vi "Tracker_171213.vi"() -> ()   [LabVIEW 2016]
uses:
  Globaltracker.vi
panel:
  in  "EXPORT 2":enum16{"RAW", "TXT", "CSV"}(ring)
  out "TotalDistanceTraveled":dbl
  out "SegmentsRecalculation":bool[](array[boolean])
  out "ForAnalysisLastRecordingPath":path
  in  "i":i32
  out "NotificationCount":i32=3
  out "Alarm":dbl caption="minutes" format="%#g"
  out "Loadedregions":picture
  out "Mousebackground":picture
  out "OutsideaSegment":dbl[](array[slide]) scale=-1.0..83.73750000001033
  out "InsideaSegment":dbl[](array[slide]) scale=-1.0..83.73750000001033
  out "TtlArray":T1(array[cluster])
  in  "Main TabControl":enum32{"Settings", "Recording", "Analysis"}(tab)
  in  "CageSegmentation":enum32{"Page 1", "Page 2"}(tab)
  out "CageSegmentation":string
  out "AssignedSegments":string
  in  "ListboxOfSegments":i32(listbox)
  in  "Border":enum32{"Page 1", "Page 2"}(tab)
  out "Border":string
  in  "Border":enum16{"8", "6", "5", "4", "3", "2", "1", "0"}(ring) caption="Number of\n segments"
  in  "StartingAngleBorder":u16=40 caption="Starting\n angle" max=360 step=1
  in  "Center":enum32{"Page 1", "Page 2"}(tab)
  in  "Center":enum16{"1", "0"}(ring) caption="Number of\n segments"
  in  "RadiusCenter":u16=40 caption="Radius \n (mm)" max=90
  out "Center":string
  in  "Midfield":enum32{"Page 1", "Page 2"}(tab)
  in  "StartingAngleMidfield":u32=40 caption="Starting\n angle" max=360 step=1
  in  "RadiusMidfield":u16=40 caption="Radius\n (mm)" max=90 step=1
  in  "Midfield":enum16{"4", "3", "2", "1", "0"}(ring) caption="Number of\n segments"
  out "Midfiled":string
  out "SettingsDisplay":picture
  out "?":picture
  in  "KeyboardShortcuts":enum32{"Page 1", "Page 2"}(tab)
  out "KeyboardShortcuts":string
  out "_Assigning Buttons_":bool
  in  "KeyBoardShortCuts":bool
  in  "Notifications":enum32{"Page 1", "Page 2"}(tab)
  out "Notifications":string
  out "Notification":bool
  in  "NotificationsON":bool
  in  "FilterType":enum32{"Page 1", "Page 2"}(tab)
  out "FIlterType":string
  in  "FilterType":enum16{"No filter", "Kalman filter"}(ring)
  in  "PortSelection":enum32{"Page 1", "Page 2"}(tab)
  out "PortSelection":string
  in  "Data Port Selection":refnum<visa-resource-name>="ASRL3::INSTR"
  in  "SAVE":bool
  out "?":picture
  in  "KeyboardShortcuts":enum32{"Page 1", "Page 2"}(tab)
  in  "SegmentsMulticolumnListbox":i32(listbox)
  out "KeyboardShortcuts":string
  out "Notification":bool
  out "RecordingDisplay":picture
  in  "Cage Segments":enum32{"Page 1", "Page 2"}(tab)
  out "Segments(s)":dbl[](array[slide]) scale=-1.0..4.437500000000029
  out "Segments":bool[](array[boolean])
  out "1":string
  out "2":string
  out "3":string
  out "4":string
  out "5":string
  out "6":string
  out "7":string
  out "8":string
  out "9":string
  out "10\n10":string
  out "11":string
  out "12":string
  out "13":string
  out "CageSegments":string
  in  "Cage orientation swap":bool caption="Swap coords"
  in  "RecordingTab":enum32{"Page 1", "Page 2"}(tab)
  in  "Stop Button":bool
  in  "Start":bool
  in  "Trace length (s)":dbl(slide) scale=0.0..10.0
  in  "DisplaySegments":enum32{"Page 1", "Page 2"}(tab)
  in  "DisplaySegments":bool caption="Display Segments"
  out "DisplaySegments":string
  in  "CurrentDistanceTraveled":enum32{"Page 1", "Page 2"}(tab)
  out "Current distance\n traveled (m)":dbl(slide) scale=0.0..8.0
  out "CurrentDistanceTraveled":string
  in  "ElapsedTimeRecording":enum32{"Page 1", "Page 2"}(tab)
  out "Time1":string
  out "Time elapsed":string
  out "ElapsedTimeRecording":string
  out "Mouse speed (cm/s)":dbl(knob) scale=0.0..100.0 scale format="%#_6f"
  out "Mouse speed (cm/s)  2":dbl(graph) caption="Mouse speed plotted vs time"
  in  "LoadRecording":enum32{"Page 1", "Page 2"}(tab)
  out "FileName":string
  out "ProgressBar":u16(slide) scale=0.0..100.0
  in  "LOAD RECORDING":bool
  in  "ElapsedTimePlayback":enum32{"Page 1", "Page 2"}(tab)
  out "Time2":string
  out "ElapsedTimePlayback":string
  out "date/time":string
  in  "PlaybackControl":enum32{"Page 1", "Page 2"}(tab)
  in  "Stop Button":bool
  in  "Start/play":bool
  in  "Skip Back Button":bool
  in  "Seek Back Button":bool
  in  "Seek Forward Button":bool
  in  "Skip Forward Button":bool
  in  "Playback progress (min)":dbl(slide) min=0.0 max=24.0 scale=0.0..1.0
  out "Display Speed":dbl
  out "Playback Speed":string
  in  "RemoveButton":bool
  in  "AddButton":bool
  out "AnalysisDisplay":picture
  out "Mouse Speed plotted vs time":dbl(graph) caption="Mouse Speed Plotted vs Time"
  out "Mouse speed (cm/s)":dbl(knob) scale=0.0..100.0
  in  "DisplayOptions":enum32{"Page 1", "Page 2"}(tab)
  in  "Heat Map":bool
  in  "Trace_length (s)":dbl(slide) scale=0.0..10.0
  in  "FullTrack":bool caption="Full Track"
  in  "SegmentsOn":bool caption="Segments"
  out "DisplayOptions":string
  in  "Statistics":enum32{"Page 1", "Page 2"}(tab)
  out "Current Distance\n Traveled (m)":dbl(slide) scale=0.0..1.0 scale format="%#_6f"
  out "Total Distance Traveled (m)":dbl
  out "Average Speed (cm/s)":dbl
  out "TTL":bool
  out "Statitics":string
  in  "EXIT":bool
  out "index":i32
  out "?":picture
  in  "TimeSpentinEachSegment":enum32{"Page 1", "Page 2"}(tab)
  out "TimeSpentinEachSegment":string
  in  "TimeSpentinEachSegmentMultiListBox":i32(listbox)
  out "Heat-Map":dbl[][](graph)
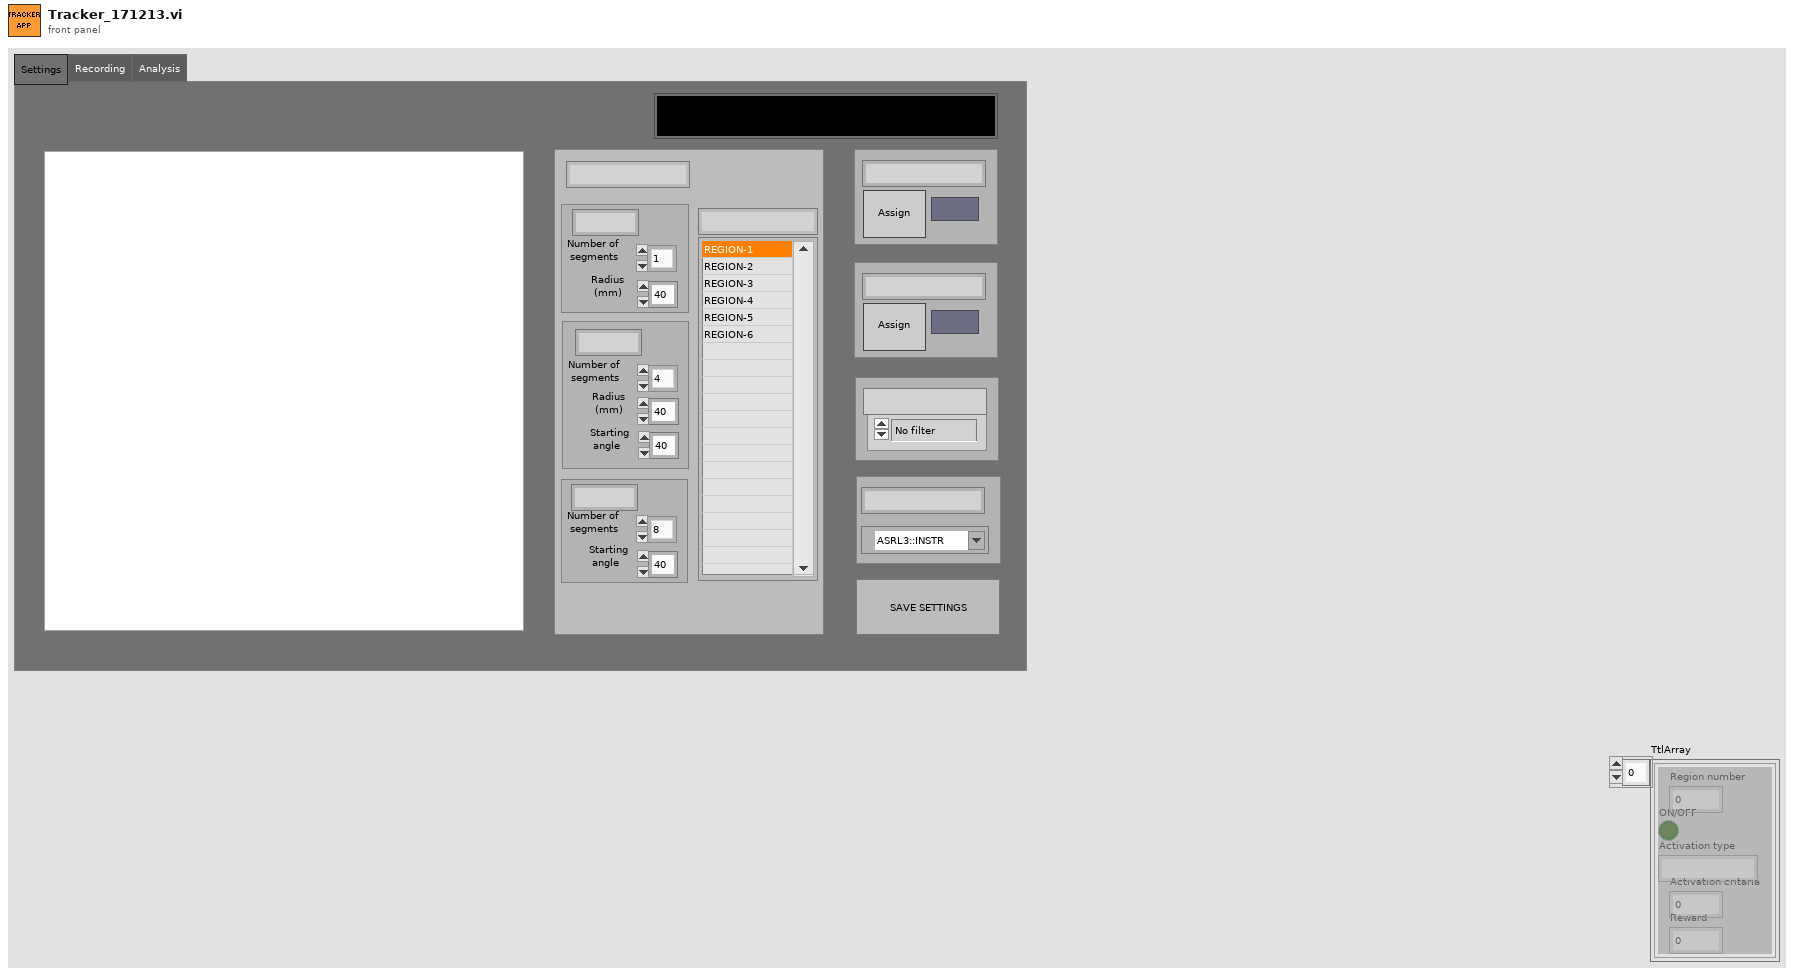
[diagram p1: front panel]
types:
  T1 = cluster{"Region number":i32, "ON/OFF":bool, "Activation type":string, "Activation critaria":i32, "Reward":i32}[]
  T2 = enum16{"No filter", "Kalman filter", "Thresholding"}
  T3 = enum8{"Enabled", "Disabled", "Disabled and Grayed Out"}
  T4 = cluster{"Starting degree of walll":u16, "RewardSystem-ON/OFF":bool, "Image Name":string, "Starting degree of walll":u16, "Starting degree of walll":u16}
  T5 = cluster{"Starting degree of walll":u16, "RewardSystem-ON/OFF":bool, "Image Name":string, "Starting degree of walll":u16, "Starting degree of walll":u16}[]
  T6 = cluster{i32, "ON-OFF":bool, "Activation":string, "ActivationCritaria":i32, "TTLActivation":i32}
  T7 = typedef "imagedata.ctl" = cluster{"image type":i32, "image depth":i32, "image":u8[], "mask":u8[], "colors":u32[], "Rectangle":cluster{"left":i16, "top":i16, "right":i16, "bottom":i16}}
  T8 = typedef "LVMouseTypeDef.ctl" = cluster{"Mouse Position":cluster{"X":i32, "Y":i32}, "Mouse Modifiers":cluster{"Button Down":bool, "Shift Mod":bool, "Menu Mod":bool, "Option Mod":bool}}
  T9 = typedef "LVDateTimeRec.ctl" = cluster{"fractional second":dbl, "second":i32, "minute":i32, "hour":i32, "day of month":i32, "month":i32, "year":i32, "day of week":i32, "day of year":i32, "DST":i32}
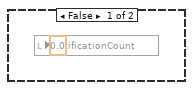
[diagram p2: hidden frame]
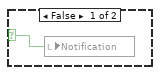
[diagram p4: hidden frame]
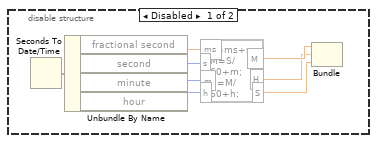
[diagram p6: hidden frame]
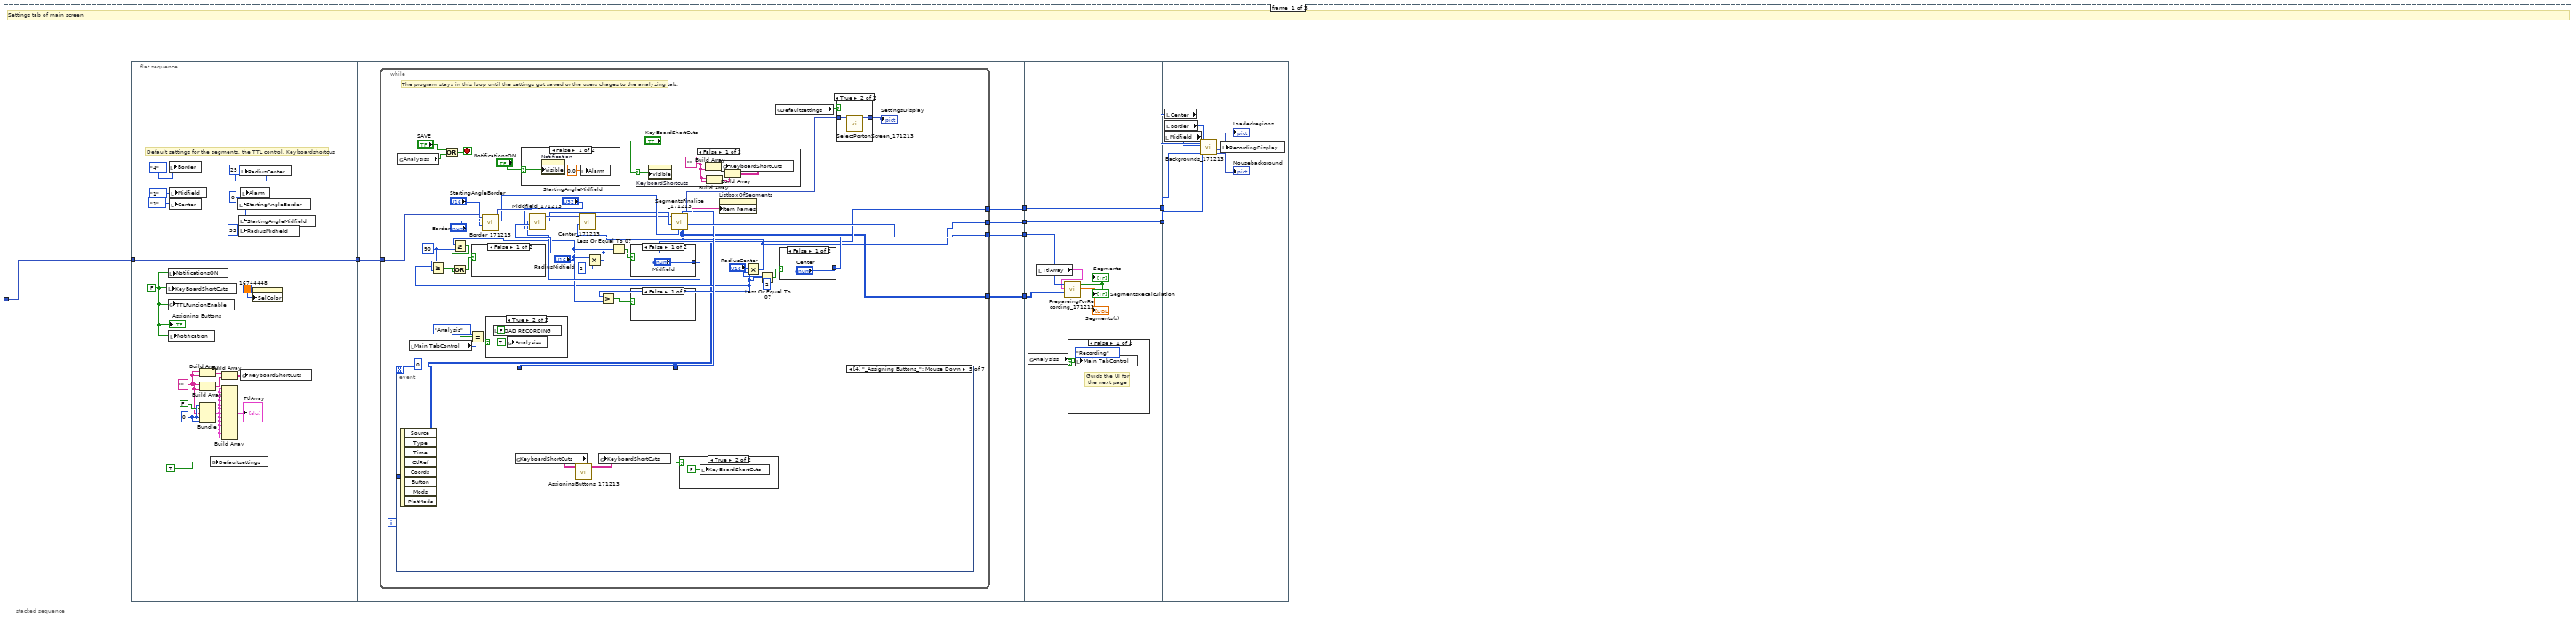
[diagram p7: hidden frame]
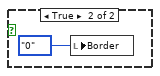
[diagram p9: hidden frame]
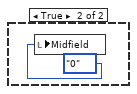
[diagram p10: hidden frame]
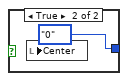
[diagram p11: hidden frame]
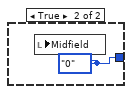
[diagram p12: hidden frame]
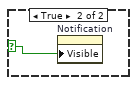
[diagram p14: hidden frame]
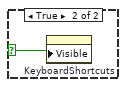
[diagram p15: hidden frame]
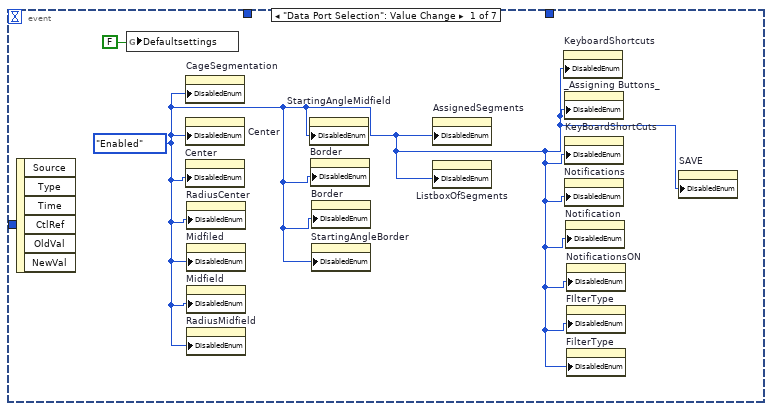
[diagram p16: hidden frame]
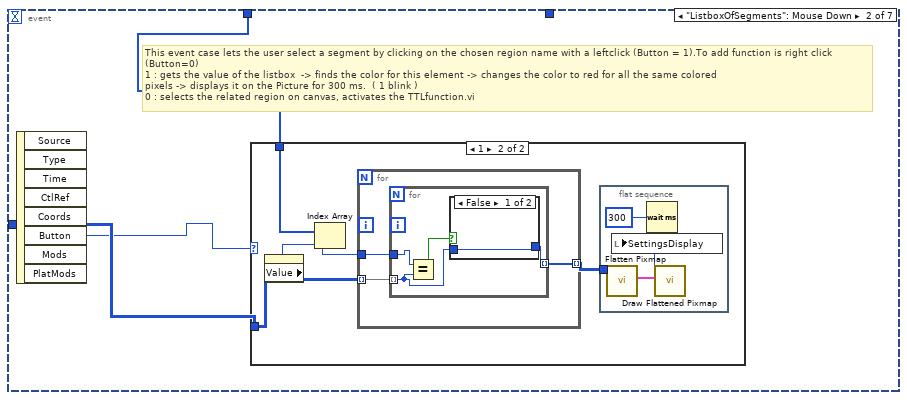
[diagram p17: hidden frame]
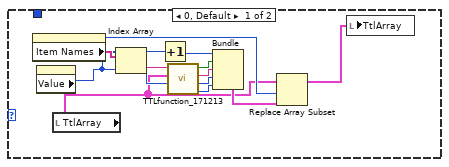
[diagram p18: hidden frame]
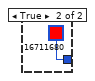
[diagram p19: hidden frame]
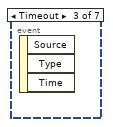
[diagram p20: hidden frame]
diagram:
  n1 = disable-structure shown="Disabled" {
    frame Disabled {
      # "This disabled notification funtion is disabled but can be put back in the \nprogram with and indicator on the screen to make the notifications \navailable in the program. It has a defined \"not moving\" speed and it \ncounts the iteration which are below that speed."
      # "ALARM\nFUNCTION"
      # "speed"
      n2 = Less Or Equal?(y=10.0) -> (x <= y?=w3:bool)  [unwired: 1 in]
      n3 = case shown="True" w3 {
        frame False {
          n4 = local write "NotificationCount"(0.0 ("alarm count")) -> ()
        }
        frame True {
          n5 = local read "NotificationCount"() -> (w8:i32)
          n6 = Increment(x=w8) -> (x+1=w5:i32)
          "NotificationCount" <- w5
          n7 = local read "Alarm"() -> (w7:dbl)
          n8 = Greater Or Equal?(x=w5, y=w7) -> (x >= y?=w6:bool)
          n9 = case shown="True" w6 {
            tunnel: w5 -> [_ w12]
            frame False {
            }
            frame True {
              n10 = To Byte Integer(number=w12) -> (8bit integer=w9:i8)
              n11 = Greater Or Equal?(x=w9, y=i8 0) -> (x >= y?=w11:bool)
              n12 = case shown="True" w11 {
                selector: w11 -> [w13 w14]
                frame False {
                  n13 = local write "Notification"(w13) -> ()
                }
                frame True {
                  "Notification" <- w14
                }
              }
            }
          }
        }
      }
    }
    frame Enabled {
    }
  }
  n14 = flat-sequence {
    tunnel: [w50] -> w1
    tunnel: w1 -> [w55]
    frame #0 {
      w15 = T3."Disabled and Grayed Out" ("Disabled")
      w49 = FALSE ("FULL TRACK")
      # "variables which have\ndefault state"
      # "Static strings : There are so many of them \nFIND option from front panel helps to find the \none\nMany Tabcontrols were used to creat blocks \non the front panel they dont have any fuctions\nexpect the Main TabControl, which is not in the\npile."
      # "These control button are never \nused to read."
      # "THIS FRAME SET THE BASIC DEFAULT STATE FOR THE PROGRAM IT RUNS ONLY ONCE AFTER THE FIRST RUN\nTHEN WE ENTER THE PROGRAM LOOP."
      # "logos"
      n15 = call "StaticStrings2_171213.vi"() -> ("Port Selection"=→"PortSelection":string, "Display"=→"DisplaySegments":string, "2"=→"2":string, "6"=→"6":string, "Midfield"=→"Midfiled":string, "7"=→"7":string, "Notifications"=→"Notifications":string, "1"=→"1":string, "9"=→"9":string)  [unwired: 7 in]
      n16 = global write "Globaltracker.vi" "Analysiss"(w49) -> ()
      n17 = global write "Globaltracker.vi" "NoFilter"(w49) -> ()
      n18 = global write "Globaltracker.vi" "Kalmanfilter"(w49) -> ()
      n19 = local write "SegmentsOn"(w49) -> ()
      n20 = local write "SAVE"(w49) -> ()
      n21 = local write "EXIT"(w49) -> ()
      n22 = global write "Globaltracker.vi" "K"(0.3 ("Threshold")) -> ()
      n23 = local write "Main TabControl"(enum32{"Settings", "Recording", "Analysis"}."Settings" ("Main TabControl")) -> ()
      n24 = local write "FilterType"(T2."Kalman filter" ("FILTER TYPE")) -> ()
      n25 = property on="Center" class="Enum (strict)"("DisabledEnum"=w15) -> ()  [unwired: 2 in, 2 out]
      n26 = property on="Center" class="Str"("DisabledEnum"=w15) -> ()  [unwired: 2 in, 2 out]
      n27 = property on="CageSegmentation" class="Str"("DisabledEnum"=w15) -> ()  [unwired: 2 in, 2 out]
      n28 = property on="RadiusCenter" class="DigNum (strict)"("DisabledEnum"=w15) -> ()  [unwired: 2 in, 2 out]
      n29 = property on="Midfiled" class="Str"("DisabledEnum"=w15) -> ()  [unwired: 2 in, 2 out]
      n30 = call "StaticTextIndicatorstoSaveSpaceonBlockdiogram_171213.vi"() -> ("8"=→"8":string, "KeyboardShortcuts"=→"KeyboardShortcuts":string, "KejyboardShortcuts2"=→"KeyboardShortcuts":string, "Statistics"=→"Statitics":string, "FilterType"=→"FIlterType":string, "CageSegments"=→"CageSegments":string, "TimeSpentinEachSegment"=→"TimeSpentinEachSegment":string, "CageSegmentation"=→"CageSegmentation":string, "AssignedSegments"=→"AssignedSegments":string, "Border"=→"Border":string, "Center"=→"Center":string, "CurrentDistanceTraveled"=→"CurrentDistanceTraveled":string, "DisplayOptions"=→"DisplayOptions":string, "3"=→"3":string, "4"=→"4":string, "ElapsedTimePlayback"=→"ElapsedTimePlayback":string, "12"=→"12":string, "13"=→"13":string, "TIme1"=→"Time1":string, "11"=→"11":string, "Time2"=→"Time2":string, "10"=→"10\n10":string, "ElapsedTimeRecording"=→"ElapsedTimeRecording":string, "5"=→"5":string)  [unwired: 4 in]
      n31 = property on="StartingAngleBorder" class="DigNum (strict)"("DisabledEnum"=w15) -> ()  [unwired: 2 in, 2 out]
      n32 = property on="Border" class="Str"("DisabledEnum"=w15) -> ()  [unwired: 2 in, 2 out]
      n33 = property on="Border" class="Enum (strict)"("DisabledEnum"=w15) -> ()  [unwired: 2 in, 2 out]
      n34 = property on="Midfield" class="Enum (strict)"("DisabledEnum"=w15) -> ()  [unwired: 2 in, 2 out]
      n35 = property on="StartingAngleMidfield" class="DigNum (strict)"("DisabledEnum"=w15) -> ()  [unwired: 2 in, 2 out]
      n36 = property on="RadiusMidfield" class="DigNum (strict)"("DisabledEnum"=w15) -> ()  [unwired: 2 in, 2 out]
      n37 = property on="ListboxOfSegments" class="LstBox (strict)"("DisabledEnum"=w15) -> ()  [unwired: 2 in, 2 out]
      n38 = property on="AssignedSegments" class="Str"("DisabledEnum"=w15) -> ()  [unwired: 2 in, 2 out]
      n39 = property on="KeyboardShortcuts" class="Str"("DisabledEnum"=w15) -> ()  [unwired: 2 in, 2 out]
      n40 = property on="KeyBoardShortCuts" class="Bool (strict)"("DisabledEnum"=w15) -> ()  [unwired: 2 in, 2 out]
      n41 = property on="_Assigning Buttons_" class="Bool"("DisabledEnum"=w15) -> ()  [unwired: 2 in, 2 out]
      n42 = property on="Notifications" class="Str"("DisabledEnum"=w15) -> ()  [unwired: 2 in, 2 out]
      n43 = property on="Notification" class="Bool"("DisabledEnum"=w15) -> ()  [unwired: 2 in, 2 out]
      n44 = call "LoadinTheStaticPictures_171213.vi"() -> ("background"=w50:picture, "logo"=→"?" →"?" →"?":picture)  [unwired: 10 in]
      n45 = property on="NotificationsON" class="Bool (strict)"("DisabledEnum"=w15) -> ()  [unwired: 2 in, 2 out]
      n46 = property on="FIlterType" class="Str"("DisabledEnum"=w15) -> ()  [unwired: 2 in, 2 out]
      n47 = property on="FilterType" class="Enum (strict)"("DisabledEnum"=w15) -> ()  [unwired: 2 in, 2 out]
      n48 = property on="SAVE" class="Bool (strict)"("DisabledEnum"=w15) -> ()  [unwired: 2 in, 2 out]
    }
    frame #1 {
      n49 = while {
        tunnel: w55 -> [w57]
        stop <- w56 stop-if-true
        # "THIS IS THE ACTUAL PROGRAM LOOP ONLY WAY TO FINISH THIS LOOP IS TO PRESS THE EXIT BUTTON. IT EXITS THE APPLICATION."
        n50 = stacked-sequence {
          tunnel: w57 -> [w61 _ _]
          tunnel: [_ _ w490] -> w56
          frame #0 {
            # "Settings tab of main screen"
            n51 = flat-sequence {
              tunnel: [w76] -> w65
              tunnel: w61 -> [w76]
              tunnel: w65 -> [w88]
              tunnel: [w87] -> w64
              tunnel: [w86] -> w63
              tunnel: [w85] -> w62
              tunnel: [w84] -> w60
              tunnel: w64 -> [w244]
              tunnel: w63 -> [w245]
              tunnel: w62 -> [w249]
              tunnel: w60 -> [w246]
              tunnel: [w245] -> w59
              tunnel: [w244] -> w58
              tunnel: w59 -> [w255]
              tunnel: w58 -> [w254]
              frame #0 {
                w69 = u16 0 ("Starting degree of walll")
                w67 = "" ("Image Name")
                w75 = u16 0 ("Starting degree of walll")
                w83 = FALSE ("RewardSystem-ON/OFF")
                # "Default settings for the segments, the TTL control, Keyboardshortcus"
                n52 = local write "KeyBoardShortCuts"(w83) -> ()
                n53 = local write "NotificationsON"(w83) -> ()
                n54 = global write "Globaltracker.vi" "TTLFuncionEnable"(w83) -> ()
                n55 = local write "Notification"(w83) -> ()
                n56 = local write "Border"(enum16{"8", "6", "5", "4", "3", "2", "1", "0"}."4" ("BORDER")) -> ()
                n57 = local write "Midfield"(enum16{"4", "3", "2", "1", "0"}."1" ("MIDFIELD")) -> ()
                n58 = local write "Center"(enum16{"1", "0"}."1" ("CENTER")) -> ()
                n59 = Build Array(w67, w67) -> (w74:string[])
                n60 = Build Array(w67, w67) -> (w72:string[])
                n61 = Bundle("Starting degree of walll"=w69, "RewardSystem-ON/OFF"=FALSE, "Image Name"=w67, "Starting degree of walll"=w69, "Starting degree of walll"=w69) -> (w70:T4)  [unwired: 1 in]
                n62 = global write "Globaltracker.vi" "Defaultsettings"(TRUE) -> ()
                n63 = Build Array(w74, w72) -> (w73:string[][])
                n64 = Build Array(w70, w70, w70, w70, w70, w70, w70, w70, w70, w70, w70, w70, w70) -> (→"TtlArray":T5)
                n65 = local write "StartingAngleBorder"(w75) -> ()
                n66 = local write "StartingAngleMidfield"(w75) -> ()
                n67 = local write "RadiusMidfield"(u16 55 ("Radius of the middfield (mm)")) -> ()
                n68 = local write "RadiusCenter"(u16 25 ("Radius of the center (mm)")) -> ()
                n69 = global write "Globaltracker.vi" "KeyboardShortCuts"(w73) -> ()
                n70 = local write "Alarm"(w75) -> ()
                n71 = property on="ListboxOfSegments" class="LstBox (strict)"("SelColor"=u32 16744448 ("color(black)")) -> ()  [unwired: 2 in, 2 out]
                "_Assigning Buttons_" <- w83
              }
              frame #1 {
                n72 = while {
                  tunnel: [w119] -> w85
                  tunnel: w88 -> [w118]
                  tunnel: [w113] -> w87
                  tunnel: [w115] -> w86
                  tunnel: [w92] -> w84
                  stop <- w108 stop-if-true
                  w96 = u16 90 ("y")
                  # "The program stays in this loop until the settings got saved or the users chages to the analyzing tab."
                  n73 = global read "Globaltracker.vi" "Analysiss"() -> (w107:bool)
                  n74 = local read "Main TabControl"() -> (w104:enum32{"Settings", "Recording", "Analysis"})
                  n75 = Greater Or Equal?(x="RadiusCenter", y=w96) -> (x >= y?=w94:bool)
                  n76 = Or(x="SAVE", y=w107) -> (x .or. y?=w108:bool)
                  n77 = Greater Or Equal?(x="RadiusMidfield", y=w96) -> (x >= y?=w98:bool)
                  n78 = Or(x=w98, y=w94) -> (x .or. y?=w97:bool)
                  n79 = Equal?(x=enum32{"Setting", "Recording", "Analysis"}."Analysis", y=w104) -> (x = y?=w106:bool)
                  n80 = case shown="False" w97 {
                    frame False {
                    }
                    frame True {
                      n81 = local write "Border"(enum16{"8", "6", "5", "4", "3", "2", "1", "0"}."0" ("BORDER")) -> ()
                    }
                  }
                  n82 = call "Border_171213.vi"("StartingAngle"="StartingAngleBorder", "Border"="Border", "InputBackground"=w118) -> ("Colors"=w124:u32[], "OutputPicture"=w127:picture)  [unwired: 7 in]
                  n83 = case shown="True" w106 {
                    frame False {
                    }
                    frame True {
                      n84 = local write "LOAD RECORDING"(FALSE ("LOAD")) -> ()
                      n85 = global write "Globaltracker.vi" "Analysiss"(TRUE ("Anal")) -> ()
                    }
                  }
                  n86 = case shown="False" "NotificationsON" {
                    selector: "NotificationsON" -> [w141 w143]
                    frame False {
                      n87 = property on="Notification" class="Bool (strict)"("Visible"=w141) -> ()  [unwired: 2 in, 2 out]
                      n88 = local write "Alarm"(0.0 ("Alarm")) -> ()
                    }
                    frame True {
                      n89 = property on="Notification" class="Bool (strict)"("Visible"=w143) -> ()  [unwired: 2 in, 2 out]
                    }
                  }
                  n90 = Multiply(x="RadiusMidfield", y=u8 2) -> (x*y=w115:u16)
                  n91 = Greater Or Equal?(x="RadiusCenter", y="RadiusMidfield") -> (x >= y?=w100:bool)
                  n92 = Less Or Equal To 0?(x="RadiusMidfield") -> (x <= 0?=w102:bool)
                  n93 = case shown="False" w102 {
                    tunnel: ["Midfield" w138] -> w103
                    frame False {
                    }
                    frame True {
                      w138 = enum16{"4", "3", "2", "1", "0"}."0" ("MIDFIELD")
                      n94 = local write "Midfield"(w138) -> ()
                    }
                  }
                  n95 = call "Middfield_171213.vi"("StartingAngle"="StartingAngleMidfield", "DiameterOfTheMidfield"=w115, "Midfield"=w103, "InputBackground"=w127) -> ("Colors"=w123:u32[], "OutputBackground"=w126:picture)  [unwired: 6 in]
                  n96 = case shown="False" w100 {
                    frame False {
                    }
                    frame True {
                      n97 = local write "Midfield"(enum16{"4", "3", "2", "1", "0"}."0" ("MIDFIELD")) -> ()
                    }
                  }
                  n98 = case shown="False" "KeyBoardShortCuts" {
                    selector: "KeyBoardShortCuts" -> [w145 w149]
                    frame False {
                      w148 = "" ("Image Name")
                      n99 = property on="KeyboardShortcuts" class="TabCtl (strict)"("Visible"=w145) -> ()  [unwired: 2 in, 2 out]
                      n100 = Build Array(w148, w148) -> (w147:string[])
                      n101 = Build Array(w148, w148) -> (w146:string[])
                      n102 = Build Array(w147, w146) -> (w144:string[][])
                      n103 = global write "Globaltracker.vi" "KeyboardShortCuts"(w144) -> ()
                    }
                    frame True {
                      n104 = property on="KeyboardShortcuts" class="TabCtl (strict)"("Visible"=w149) -> ()  [unwired: 2 in, 2 out]
                    }
                  }
                  n105 = Multiply(x="RadiusCenter", y=u8 2) -> (x*y=w113:u16)
                  n106 = Less Or Equal To 0?(x="RadiusCenter") -> (x <= 0?=w101:bool)
                  n107 = global read "Globaltracker.vi" "Defaultsettings"() -> (w91:bool)
                  n108 = case shown="False" w101 {
                    tunnel: ["Center" w136] -> w125
                    frame False {
                    }
                    frame True {
                      w136 = enum16{"1", "0"}."0" ("CENTER")
                      n109 = local write "Center"(w136) -> ()
                    }
                  }
                  n110 = call "Center_171213.vi"("DiameterOfTheCenter"=w113, "Center"=w125, "InputBackground"=w126) -> ("Colors"=w122:u32[], "OutputBackground"=w121:picture)  [unwired: 7 in]
                  n111 = call "SegmentsFinalize_171213.vi"("BorderColor"=w124, "MidfieldColor"=w123, "CenterColor"=w122, "InputBackground"=w121) -> ("TotalNumberOfSegments"=w119:i32, "RegionNameList"=w120:string[], "Outputbackground"=w90:picture, "OutputPixmapforEvents"=w92:u32[][], "ColorArrayforEvents"=w116:u32[])  [unwired: 3 in]
                  n112 = event shown="[4] \"_Assigning Buttons_\": Mouse Down" {
                    selector: _ -> [_ _ _ _ _ _ _]
                    dyn-events: _ -> [_ _ _ _ _ _ _]
                    timeout: 0 -> [_ _ _ _ _ _ _]
                    tunnel: w92 -> [_ w154 _ w186 _ _ _]
                    tunnel: w116 -> [_ _ _ w185 _ _ _]
                    tunnel: w116 -> [_ w153 _ _ _ _ _]
                    event "Data Port Selection": Value Change {
                      w150 = T3."Enabled" ("Disabled")
                      n113 = event-data() -> ()  [unwired: 1 in, 6 out]
                      n114 = global write "Globaltracker.vi" "Defaultsettings"(FALSE) -> ()
                      n115 = property on="CageSegmentation" class="Str"("DisabledEnum"=w150) -> ()  [unwired: 2 in, 2 out]
                      n116 = property on="Center" class="Str"("DisabledEnum"=w150) -> ()  [unwired: 2 in, 2 out]
                      n117 = property on="Center" class="Enum (strict)"("DisabledEnum"=w150) -> ()  [unwired: 2 in, 2 out]
                      n118 = property on="RadiusCenter" class="DigNum (strict)"("DisabledEnum"=w150) -> ()  [unwired: 2 in, 2 out]
                      n119 = property on="Midfiled" class="Str"("DisabledEnum"=w150) -> ()  [unwired: 2 in, 2 out]
                      n120 = property on="Midfield" class="Enum (strict)"("DisabledEnum"=w150) -> ()  [unwired: 2 in, 2 out]
                      n121 = property on="RadiusMidfield" class="DigNum (strict)"("DisabledEnum"=w150) -> ()  [unwired: 2 in, 2 out]
                      n122 = property on="StartingAngleMidfield" class="DigNum (strict)"("DisabledEnum"=w150) -> ()  [unwired: 2 in, 2 out]
                      n123 = property on="Border" class="Str"("DisabledEnum"=w150) -> ()  [unwired: 2 in, 2 out]
                      n124 = property on="Border" class="Enum (strict)"("DisabledEnum"=w150) -> ()  [unwired: 2 in, 2 out]
                      n125 = property on="StartingAngleBorder" class="DigNum (strict)"("DisabledEnum"=w150) -> ()  [unwired: 2 in, 2 out]
                      n126 = property on="AssignedSegments" class="Str"("DisabledEnum"=w150) -> ()  [unwired: 2 in, 2 out]
                      n127 = property on="ListboxOfSegments" class="LstBox (strict)"("DisabledEnum"=w150) -> ()  [unwired: 2 in, 2 out]
                      n128 = property on="KeyboardShortcuts" class="Str"("DisabledEnum"=w150) -> ()  [unwired: 2 in, 2 out]
                      n129 = property on="_Assigning Buttons_" class="Bool"("DisabledEnum"=w150) -> ()  [unwired: 2 in, 2 out]
                      n130 = property on="KeyBoardShortCuts" class="Bool (strict)"("DisabledEnum"=w150) -> ()  [unwired: 2 in, 2 out]
                      n131 = property on="Notifications" class="Str"("DisabledEnum"=w150) -> ()  [unwired: 2 in, 2 out]
                      n132 = property on="Notification" class="Bool"("DisabledEnum"=w150) -> ()  [unwired: 2 in, 2 out]
                      n133 = property on="NotificationsON" class="Bool (strict)"("DisabledEnum"=w150) -> ()  [unwired: 2 in, 2 out]
                      n134 = property on="FIlterType" class="Str"("DisabledEnum"=w150) -> ()  [unwired: 2 in, 2 out]
                      n135 = property on="FilterType" class="Enum (strict)"("DisabledEnum"=w150) -> ()  [unwired: 2 in, 2 out]
                      n136 = property on="SAVE" class="Bool (strict)"("DisabledEnum"=w150) -> ()  [unwired: 2 in, 2 out]
                    }
                    event "ListboxOfSegments": Mouse Down {
                      # "This event case lets the user select a segment by clicking on the chosen region name with a leftclick (Button = 1).To add function is right click \n(Button=0)\n1 : gets the value of the listbox  -> finds the color for this element -> changes the color to red for all the same colored\npixels -> displays it on the Picture for 300 ms.  ( 1 blink ) \n0 : selects the related region on canvas, activates the TTLfunction.vi"
                      n137 = event-data() -> ("Button"=w152:u16)  [unwired: 1 in, 7 out]
                      n138 = case shown="1" w152 {
                        tunnel: w154 -> [_ w167]
                        tunnel: w153 -> [_ w166]
                        frame 0, Default {
                          n139 = property on="ListboxOfSegments" class="LstBox (strict)"() -> ("Item Names"=w165:string[])  [unwired: 2 in, 2 out]
                          n140 = property on="ListboxOfSegments" class="LstBox (strict)"() -> ("Value"=w157:i32)  [unwired: 2 in, 2 out]
                          n141 = local read "TtlArray"() -> (w156:T1)
                          n142 = Index Array(array=w165, index=w157) -> (element=w164:string)
                          n143 = Increment(x=w157) -> (x+1=w158:i32)
                          n144 = call "TTLfunction_171213.vi"("RegionClicked"=w157, "TTLArray"=w156, "INPUT STRING"=w164) -> ("TTLActivation"=w160:i32, "ActivationCritaria"=w161:i32, "Activation"=w162:string, "ON-OFF"=w163:bool)  [unwired: 5 in]
                          n145 = Bundle(w158, "ON-OFF"=w163, "Activation"=w162, "ActivationCritaria"=w161, "TTLActivation"=w160) -> (w159:T6)  [unwired: 1 in]
                          n146 = Replace Array Subset(array=w156, new element=w159, index=w157) -> (w155:T1)
                          n147 = local write "TtlArray"(w155) -> ()
                        }
                        frame 1 {
                          n148 = property on="ListboxOfSegments" class="LstBox (strict)"() -> ("Value"=w170:i32)  [unwired: 2 in, 2 out]
                          n149 = Index Array(array=w166, index=w170) -> (element=w169:u32)
                          n150 = for {
                            tunnel: w167 -> [w177] mode=indexing
                            tunnel: w169 -> [w176]
                            tunnel: [w175] -> w168 mode=indexing
                            n151 = for {
                              tunnel: w177 -> [w179] mode=indexing
                              tunnel: w176 -> [w180]
                              tunnel: [w178] -> w175 mode=indexing
                              n152 = Equal?(x=w180, y=w179) -> (x = y?=w181:bool)
                              n153 = case shown="False" w181 {
                                tunnel: [w182 u32 16711680 ("color(black)")] -> w178
                                tunnel: w179 -> [w182 _]
                                frame False {
                                }
                                frame True {
                                }
                              }
                            }
                          }
                          n154 = flat-sequence {
                            tunnel: w168 -> [w174]
                            frame #0 {
                              n155 = call <vilib>:"Flatten Pixmap.vi"("24-bit pixmap"=w174) -> ("image data"=w173:T7)  [unwired: 10 in]
                              n156 = Wait (ms)(milliseconds to wait=u32 300) -> ()  [unwired: 1 out]
                              n157 = call <vilib>:"Draw Flattened Pixmap.vi"("image data"=w173) -> ("new picture"=w172:picture)  [unwired: 8 in]
                              n158 = local write "SettingsDisplay"(w172) -> ()
                            }
                          }
                        }
                      }
                    }
                    event Timeout {
                      n159 = event-data() -> ()  [unwired: 1 in, 3 out]
                    }
                    event "SettingsDisplay": Mouse Down {
                      # "This event case lets the user select a segment by clicking on the chosen sector with a leftclick (Button=1). to add function is right click (Button =0).\n 1 : gets the mouse coordinate cuts the circle first  -> finds which color the mouse is on -> changes the color to red for all the same colored\npixels -> displays it on the Picture for 200 ms.  ( 1 blink can be changed )\n 0 : selects the related region on the from the Listbox, activates the TTLfunction.vi"
                      n160 = event-data() -> ("Button"=w184:u16)  [unwired: 1 in]
                      n161 = case shown="0, Default" w184 {
                        tunnel: w186 -> [_ w204]
                        tunnel: w185 -> [_ w200]
                        frame 0, Default {
                          n162 = property on="ListboxOfSegments" class="LstBox (strict)"() -> ("Value"=w196:i32)  [unwired: 2 in, 2 out]
                          n163 = property on="ListboxOfSegments" class="LstBox (strict)"() -> ("Item Names"=w188:string[])  [unwired: 2 in, 2 out]
                          n164 = local read "TtlArray"() -> (w197:T1)
                          n165 = Index Array(array=w188, index=w196) -> (element=w189:string)
                          n166 = Increment(x=w196) -> (x+1=w195:i32)
                          n167 = call "TTLfunction_171213.vi"("RegionClicked"=w196, "TTLArray"=w197, "INPUT STRING"=w189) -> ("TTLActivation"=w193:i32, "ActivationCritaria"=w192:i32, "Activation"=w191:string, "ON-OFF"=w190:bool)  [unwired: 5 in]
                          n168 = Bundle(w195, "ON-OFF"=w190, "Activation"=w191, "ActivationCritaria"=w192, "TTLActivation"=w193) -> (w194:T6)  [unwired: 1 in]
                          n169 = Replace Array Subset(array=w197, new element=w194, index=w196) -> (w187:T1)
                          n170 = local write "TtlArray"(w187) -> ()
                        }
                        frame 1 {
                          n171 = property on="SettingsDisplay" class="Pict"() -> ("Mouse"=w202:T8)  [unwired: 2 in, 2 out]
                          n172 = Unbundle(w202) -> ("Mouse Position"=w201:cluster{"X":i32, "Y":i32})  [unwired: 1 out]
                          n173 = Unbundle(w201) -> ("X"=w198:i32, "Y"=w199:i32)
                          n174 = Index Array(array=w204, index (row)=w199, index (col)=w198) -> (element=w203:u32)
                          n175 = for {
                            tunnel: w204 -> [w214] mode=indexing
                            tunnel: [w213] -> w205 mode=indexing
                            tunnel: w203 -> [w212]
                            tunnel: w203 -> [w211]
                            tunnel: w200 -> [w210]
                            n176 = for {
                              tunnel: w214 -> [w219] mode=indexing
                              tunnel: [w218] -> w213 mode=indexing
                              tunnel: w212 -> [w217]
                              tunnel: w211 -> [w216]
                              tunnel: w210 -> [w215]
                              n177 = Equal?(x=w217, y=w219) -> (x = y?=w220:bool)
                              n178 = case shown="True" w220 {
                                tunnel: [w221 u32 16711680 ("color(black)")] -> w218
                                tunnel: w219 -> [w221 _]
                                tunnel: w216 -> [_ w223]
                                tunnel: w215 -> [_ w222]
                                frame False {
                                }
                                frame True {
                                n179 = Search 1D Array(1D array=w222, element=w223) -> (index of element=w224:i32)  [unwired: 1 in]
                                n180 = property on="ListboxOfSegments" class="LstBox (strict)"("Value"=w224) -> ()  [unwired: 2 in, 2 out]
                                }
                              }
                            }
                          }
                          n181 = call <vilib>:"Flatten Pixmap.vi"("24-bit pixmap"=w205) -> ("image data"=w206:T7)  [unwired: 10 in]
                          n182 = flat-sequence {
                            tunnel: w206 -> [w209]
                            frame #0 {
                              n183 = call <vilib>:"Draw Flattened Pixmap.vi"("image data"=w209) -> ("new picture"=w207:picture)  [unwired: 8 in]
                              n184 = local write "SettingsDisplay"(w207) -> ()
                              n185 = Wait (ms)(milliseconds to wait=u32 200) -> ()  [unwired: 1 out]
                            }
                          }
                        }
                      }
                    }
                    event "_Assigning Buttons_": Mouse Down {
                      n186 = event-data() -> ()  [unwired: 1 in, 8 out]
                      n187 = global read "Globaltracker.vi" "KeyboardShortCuts"() -> (w226:string[][])
                      n188 = call "AssigningButtons_171213.vi"("Input"=w226) -> ("Cancel Button 2"=w228:bool, "outputarray"=w227:string[][])  [unwired: 9 in]
                      n189 = global write "Globaltracker.vi" "KeyboardShortCuts"(w227) -> ()
                      n190 = case shown="True" w228 {
                        frame False {
                          n191 = local write "KeyBoardShortCuts"(TRUE ("Assigning Buttons")) -> ()
                        }
                        frame True {
                          n192 = local write "KeyBoardShortCuts"(FALSE ("Assigning Buttons")) -> ()
                        }
                      }
                    }
                    event "FilterType": Value Change {
                      # "This event case deals with the filter type for the display of the data stream. It asks the user with a custom made prompt up\nwindow to set the coefficient for the chosen filter.  This number also can be the coefficient for the quoaternion rotation ?"
                      n193 = event-data() -> ("NewVal"=w231:enum16{"No filter", "Kalman filter"})  [unwired: 1 in, 5 out]
                      n194 = case shown="\"Kalman filter\"" w231 {
                        frame "No filter", Default {
                          n195 = global write "Globaltracker.vi" "NoFilter"(TRUE ("Nofilter")) -> ()
                        }
                        frame "Kalman filter" {
                          n196 = call "Kalmancoefficient_171213.vi"() -> ("K"=w233:dbl)  [unwired: 17 in, 2 out]
                          n197 = global write "Globaltracker.vi" "Kalmanfilter"(TRUE ("Nofilter")) -> ()
                          n198 = global write "Globaltracker.vi" "K"(w233) -> ()
                          n199 = global write "Globaltracker.vi" "NoFilter"(FALSE ("Nofilter")) -> ()
                        }
                      }
                    }
                    event "Notification": Mouse Down {
                      # "Converting from minutes to actual iteration number."
                      # "This event case is for the notifications. NOT IN FULL FUNCTION NOW\n This function has to be further developed with additional options for useres.\nNow it would watch the speed of the mouse if it is under a certain value for a given time period then it actives a \"heads\nups\" indicator on the screen."
                      n200 = event-data() -> ()  [unwired: 1 in, 8 out]
                      n201 = call "Alarm_171213.vi"() -> ("CANCEL"=w236:bool, "minutes"=w241:dbl)  [unwired: 16 in, 2 out]
                      n202 = case shown="False" w236 {
                        frame False {
                          n203 = local write "NotificationsON"(TRUE ("_Alarm")) -> ()
                        }
                        frame True {
                          n204 = local write "NotificationsON"(FALSE ("_Alarm")) -> ()
                        }
                      }
                      n205 = Multiply(x=60.0, y=w241) -> (x*y=w240:dbl)
                      n206 = Multiply(x=80.0, y=w240) -> (x*y=→"Alarm":dbl)
                    }
                  }
                  n207 = property on="ListboxOfSegments" class="LstBox (strict)"("Item Names"=w120) -> ()  [unwired: 2 in, 2 out]
                  n208 = case shown="True" w91 {
                    tunnel: w90 -> [w130 w132]
                    tunnel: [w130 w131] -> w89
                    frame False {
                    }
                    frame True {
                      n209 = call "SelectPortonScreen_171213.vi"("input"=w132) -> ("output"=w131:picture)  [unwired: 10 in]
                    }
                  }
                  "SettingsDisplay" <- w89
                }
              }
              frame #2 {
                n210 = global read "Globaltracker.vi" "Analysiss"() -> (w248:bool)
                n211 = local read "TtlArray"() -> (w247:T1)
                n212 = call "PrepareingForRecording_171213.vi"("OutputPixmapforCalculations"=w246, "TTLArray"=w247, "TotalNumberOfSegments"=w249) -> ("Segments(s)"=→"Segments(s)":dbl[], "Segments"=→"Segments" →"SegmentsRecalculation":bool[])  [unwired: 7 in]
                n213 = case shown="False" w248 {
                  frame False {
                    # "Guids the UI for\n the next page"
                    n214 = local write "Main TabControl"(enum32{"Settings", "Recording", "Analysis"}."Recording" ("Main TabControl")) -> ()
                  }
                  frame True {
                    n215 = local write "LOAD RECORDING"(FALSE ("LOAD")) -> ()
                  }
                }
              }
              frame #3 {
                n216 = local read "Midfield"() -> (w259:enum16{"4", "3", "2", "1", "0"})
                n217 = local read "Center"() -> (w260:enum16{"1", "0"})
                n218 = local read "Border"() -> (w258:enum16{"8", "6", "5", "4", "3", "2", "1", "0"})
                n219 = call "Backgrounds_171213.vi"("CENTER"=w260, "DiameterOfTheMidfield"=w255, "DiaMeterOfTheCenter"=w254, "MIDFIELD"=w259, "BORDER"=w258) -> ("OutputMouseBackground"=→"Mousebackground":picture, "NumberedOutput"=w256:picture)  [unwired: 5 in]
                "Loadedregions" <- w256
                n220 = local write "RecordingDisplay"(w256) -> ()
              }
            }
          }
          frame #1 {
            # "Recording tab of main screen"
            n221 = global read "Globaltracker.vi" "Analysiss"() -> (w261:bool)
            n222 = case shown="False" w261 {
              frame False {
                n223 = call "Cage_setup_171213.vi"("Close port? (T)"=FALSE ("Close port"), "VISA resource name"="Data Port Selection") -> ("Record_flag"=w263:refnum<notifier>, "error"=w265:bool, "ReadStatus"=w264:refnum<notifier>, "VISA resource name out"=w266:refnum<visa-resource-name>)  [unwired: 3 in]
                n224 = case shown="False" w265 {
                  selector: w265 -> [_ w485]
                  tunnel: w264 -> [w283 _]
                  tunnel: w263 -> [w282 _]
                  tunnel: w266 -> [w281 _]
                  frame False {
                    n225 = flat-sequence {
                      tunnel: [w305] -> w291
                      tunnel: [w306] -> w290
                      tunnel: [w307] -> w289
                      tunnel: [w309] -> w288
                      tunnel: w283 -> [w307]
                      tunnel: w282 -> [w306]
                      tunnel: w281 -> [w305]
                      tunnel: [w304] -> w279
                      tunnel: [w303] -> w277
                      tunnel: [w299] -> w276
                      tunnel: [i32[] [] ("Y out")] -> w275
                      tunnel: [w297] -> w274
                      tunnel: [w296] -> w273
                      tunnel: [w295] -> w272
                      tunnel: [w294] -> w271
                      tunnel: [w293] -> w270
                      tunnel: [w293] -> w269
                      tunnel: [w292] -> w268
                      tunnel: w291 -> [w330]
                      tunnel: w290 -> [w335]
                      tunnel: w289 -> [w334]
                      tunnel: w288 -> [w333]
                      tunnel: [w319] -> w287
                      tunnel: [w332] -> w286
                      tunnel: [w320] -> w285
                      tunnel: [w331] -> w284
                      tunnel: [w329] -> w280
                      tunnel: w279 -> [w328]
                      tunnel: [w327] -> w278
                      tunnel: w277 -> [w327]
                      tunnel: w276 -> [w326]
                      tunnel: w275 -> [w325]
                      tunnel: w274 -> [w324]
                      tunnel: w273 -> [w323]
                      tunnel: w272 -> [w322]
                      tunnel: w271 -> [w321]
                      tunnel: w270 -> [w320]
                      tunnel: w269 -> [w318]
                      tunnel: w268 -> [w319]
                      tunnel: w287 -> [w462]
                      tunnel: w286 -> [_]
                      tunnel: w285 -> [w461]
                      tunnel: w284 -> [w466]
                      tunnel: w280 -> [w463]
                      tunnel: w278 -> [w464]
                      frame #0 {
                        w302 = 0.0 ("SUM PATH ( m)")
                        w310 = FALSE ("VISIBLE REGIONS")
                        # "Set most the used displayes and variable to default"
                        n226 = while {
                          tunnel: ["Start"] -> w309
                          tunnel: [w313] -> w304
                          tunnel: [w313] -> w303
                          stop <- w314 stop-if-true
                          # "Allows the user to go back to\nsettings before pressing \nRECORD"
                          n227 = local read "Main TabControl"() -> (w317:enum32{"Settings", "Recording", "Analysis"})
                          n228 = Equal?(x=w317, y=enum32{"Setting", "Recording", "Analysis"}."Setting") -> (x = y?=w313:bool)
                          n229 = global write "Globaltracker.vi" "TrackerDisabled"(w313) -> ()
                          n230 = Or(x="Start", y=w313) -> (x .or. y?=w314:bool)
                        }
                        n231 = local write "Mouse speed (cm/s)"(w302) -> ()
                        n232 = local write "NotificationCount"(w302) -> ()
                        n233 = local write "i"(w302) -> ()
                        n234 = global write "Globaltracker.vi" "TTLSignalActive"(w310) -> ()
                        n235 = property on="Mouse speed (cm/s)  2" class="WFChart (strict)"("History Data"=dbl[] []) -> ()  [unwired: 2 in, 2 out]
                        n236 = local write "Notification"(w310) -> ()
                        n237 = global write "Globaltracker.vi" "Done"(w310) -> ()
                        n238 = local write "Time elapsed"("00:00:00.000" ("date/time string")) -> ()
                        n239 = local read "Segments(s)"() -> (→"InsideaSegment" →"OutsideaSegment":dbl[])
                        n240 = Seconds To Date/Time(time stamp (now)=timestamp(0 s since 1904-01-01) ("current time"), to UTC (F)=TRUE) -> (date time rec=w299:T9)
                        n241 = local read "Mousebackground"() -> (w297:picture)
                        n242 = local read "Loadedregions"() -> (w296:picture)
                        n243 = local read "Segments(s)"() -> (w294:dbl[])
                        n244 = local read "Segments"() -> (w295:bool[])
                        n245 = call "Get_temporary_save_path_171213.vi"() -> ("Temporary file output path"=w293:path, "date/time string"=w292:string)  [unwired: 2 in]
                        "TotalDistanceTraveled" <- w302
                        "Current distance\n traveled (m)" <- w302
                      }
                      frame #1 {
                        n246 = case shown="False" w328 {
                          tunnel: w335 -> [w352 w460]
                          tunnel: w334 -> [w351 _]
                          tunnel: w333 -> [w350 _]
                          tunnel: [w349 w460] -> w332
                          tunnel: [w348 w459] -> w331
                          tunnel: w330 -> [w346 w459]
                          tunnel: [w344 w458] -> w329
                          tunnel: w326 -> [w342 _]
                          tunnel: w325 -> [w341 _]
                          tunnel: w324 -> [w340 _]
                          tunnel: w323 -> [w339 _]
                          tunnel: w322 -> [w338 _]
                          tunnel: w321 -> [w337 _]
                          tunnel: w318 -> [w336 _]
                          frame False {
                            # "This main loop is the actual recording period. It terminates if the STOP button is pressed or the Tracker is not connected or does not send the signals.  There is a saving procedure (Save_incrementally.vi)  in this loop which save every data without any additional calculations. \nFurthermore it checks a random ( i = 88)  signal  is correct or not from the tracker if it is not correct the loop terminates and the program displays an error message. (TrackerDisabled case structure)\nOtherwise the streamed data is going to be represented on the screen. On the screen the program only displays every third iteration in order to\ngain speed to the program and it is still over 26 fps display which seems continiuos for a human eye. (other case structure)"
                            n247 = global read "Globaltracker.vi" "TTLFuncionEnable"() -> (w345:bool)
                            n248 = local read "KeyBoardShortCuts"() -> (w343:bool)
                            n249 = local write "Start/play"(FALSE ("Start/play")) -> ()
                            n250 = case shown="True" w345 {
                              tunnel: w346 -> [_ w353]
                              frame False {
                              }
                              frame True {
                                n251 = call "TrackerTTLsignal_171213.vi"("Serial Port"=w353) -> ()  [unwired: 11 in]
                              }
                            }
                            n252 = case shown="True" w343 {
                              frame False {
                              }
                              frame True {
                                n253 = call "Keyboardshortcuts_171213.vi"() -> ()  [unwired: 12 in]
                              }
                            }
                            n254 = while {
                              shift-right: [w399] -> w344
                              shift-left: w337 -> [w410]
                              shift-right: [w359] -> _
                              shift-left: w338 -> [w360]
                              shift-right: [w409] -> _
                              shift-left: w337 -> [w408]
                              shift-right: [w406] -> _
                              shift-left: w337 -> [w407]
                              shift-right: [w404] -> _
                              shift-left: w342 -> [w405]
                              shift-right: [w398] -> _
                              shift-left: w341 -> [w367]
                              shift-right: [w396] -> _
                              shift-left: w341 -> [w397]
                              tunnel: w346 -> [w384]
                              tunnel: w352 -> [w393]
                              tunnel: w351 -> [w392]
                              tunnel: w350 -> [w390]
                              tunnel: [w391] -> w349
                              tunnel: [w389] -> w348
                              tunnel: [w366] -> _
                              tunnel: w340 -> [w365]
                              tunnel: w339 -> [w364]
                              tunnel: w336 -> [w363]
                              i -> [w356]
                              stop <- w366 stop-if-true
                              w362 = u32 12 ("milliseconds to wait")
                              n255 = call "Stream_data_171213.vi"("VISA resource name in"=w384, "Play / Pause"=w390, "Notifier in"=w392) -> ("read buffer"=w381:string, "VISA Refnum out"=w389:refnum<visa-resource-name>)  [unwired: 5 in, 2 out]
                              n256 = Increment(x=w362) -> (x+1=w361:u32)
                              n257 = case shown="True" w390 {
                                tunnel: w393 -> [w420 w423]
                                tunnel: [w420 w421] -> w391
                                frame False {
                                }
                                frame True {
                                n258 = Send Notification(notification=1, notifier=w423) -> (notifier out=w421:refnum<notifier>)  [unwired: 1 in, 1 out]
                                }
                              }
                              n259 = call "Time_171213.vi"("TimeIn"=w405) -> (2:"TimeOut"=→"Time elapsed":string, 3:"TimeOut"=w404:T9)  [unwired: 9 in]
                              n260 = call "Decode_RAW_to_DEC_171213.vi"("read buffer"=w381) -> ("DEC SGL output"=w357:sgl[][])
                              n261 = Wait (ms)(milliseconds to wait=w361) -> ()  [unwired: 1 out]
                              n262 = call "Save_incrementally_171213.vi"("Temporary file output path"=w363, "Play / Pause"=TRUE, "Sensor read input"=w357, "Loop iteration"=w356, "Loop speed in ms"=w362, "Save every N seconds"=u32 5) -> ()  [unwired: 8 in, 2 out]
                              n263 = call "RecordingDisplayCalculations_171213.vi"("i"=w356, "DeCOutput"=w357) -> ("Rel Y"=w354:sgl, "Rel X"=w355:sgl, "Mouse angle"=w374:sgl)  [unwired: 7 in]
                              n264 = Empty String/Path?(string/path=w381) -> (empty?=w378:bool)
                              n265 = local read "TotalDistanceTraveled"() -> (w387:dbl)
                              n266 = global read "Globaltracker.vi" "NoFilter"() -> (w382:bool)
                              n267 = case shown="False" w382 {
                                tunnel: w355 -> [w417 w418]
                                tunnel: w354 -> [w416 w419]
                                tunnel: w356 -> [w415 _]
                                tunnel: [w414 w418] -> w386
                                tunnel: [w413 w419] -> w385
                                frame False {
                                n268 = call "KalmanforRelX,Y,angle_171213.vi"("i"=w415, "RelY"=w416, "RelX"=w417) -> ("nextY"=w413:dbl, "nextX"=w414:dbl)  [unwired: 6 in, 1 out]
                                }
                                frame True {
                                }
                              }
                              n269 = Equal?(x=w356, y=88) -> (x = y?=w379:bool)
                              n270 = And(x=w379, y=w378) -> (x .and. y?=w377:bool)
                              n271 = case shown="True" w377 {
                                frame False {
                                }
                                frame True {
                                n272 = One Button Dialog(message="ERROR:Tracker is not connected") -> ()  [unwired: 1 in, 1 out]
                                n273 = global write "Globaltracker.vi" "TrackerDisabled"(TRUE ("helping")) -> ()
                                }
                              }
                              n274 = call "DisplacementCalc_171213.vi"("TotalDistanceTraveledInput"=w387, "i"=w356, "Y"=w385, "X"=w386) -> ("Speed"=w368:dbl, "TotalDistanceTraveledOutput"=w373:dbl)  [unwired: 6 in]
                              n275 = local write "TotalDistanceTraveled"(w373) -> ()
                              n276 = Increment(x=w373) -> (x+1=w370:dbl)
                              n277 = call "TransformTo360_171213.vi"("nextY"=w385, "nextX"=w386) -> ("X"=w395:i32, "Y"=w394:i32)  [unwired: 8 in]
                              n278 = Round Toward +Infinity(x=w370) -> (ceil(x): smallest int >= x=w371:dbl)
                              n279 = Multiply(x=4.0, y=w371) -> (x*y=w369:dbl)
                              n280 = call "TheCoordinateColor_171213.vi"("InputSegments"=w360, "X"=w395, "Y"=w394, "InputSegments(s)"=w410) -> ("MATCH index"=w400:i32, "Outputsegments"=w359:bool[], "OutputSegmens(s)"=w399:dbl[])  [unwired: 5 in]
                              n281 = property on="Current distance\n traveled (m)" class="Slide (strict)"("Scale.Maximum"=w369) -> ()  [unwired: 2 in, 2 out]
                              n282 = call "TTLsignalactivation_171213.vi"("Outside in"=w407, "InputcurrentSegement"=w359, "Inside in"=w408, "InputpriviousSegment"=w360, "MATCH index"=w400) -> ("Inside out"=w409:dbl[], "Outside out"=w406:dbl[])  [unwired: 5 in]
                              n283 = Quotient & Remainder(x=w356, y=3.0 ("x")) -> (x-y*floor(x/y)=w403:dbl)  [unwired: 1 out]
                              n284 = Equal To 0?(x=w403) -> (x = 0?=w402:bool)
                              n285 = case shown="True" w402 {
                                tunnel: w368 -> [_ w457]
                                tunnel: w359 -> [_ w456]
                                tunnel: w399 -> [_ w454]
                                tunnel: w373 -> [_ w455]
                                tunnel: w365 -> [_ w452]
                                tunnel: w364 -> [_ w451]
                                tunnel: w395 -> [_ w450]
                                tunnel: w394 -> [_ w449]
                                tunnel: w374 -> [_ w429]
                                tunnel: w368 -> [_ w447]
                                tunnel: w367 -> [w425 w446]
                                tunnel: [w425 w445] -> w398
                                tunnel: w397 -> [w424 w444]
                                tunnel: [w424 w443] -> w396
                                frame False {
                                }
                                frame True {
                                n286 = Subtract(x=w429, y=sgl 180.0) -> (x-y=w431:sgl)
                                n287 = Less Or Equal To 0?(x=w429) -> (x <= 0?=w433:bool)
                                n288 = Add(x=w429, y=sgl 180.0) -> (x+y=w428:sgl)
                                n289 = Select(t=w428, s=w433, f=w431) -> (s? t:f=w432:sgl)
                                n290 = local write "Segments"(w456) -> ()
                                n291 = Select(t=w432, s="Cage orientation swap", f=w429) -> (s? t:f=w434:sgl)
                                n292 = Multiply(x="Trace length (s)", y=26.666) -> (x*y=w437:dbl)
                                n293 = global write "Globaltracker.vi" "Cage orientation swapped"("Cage orientation swap") -> ()
                                n294 = Round To Nearest(number=w437) -> (nearest integer value=w435:dbl)
                                n295 = global read "Globaltracker.vi" "KeyboardShortCuts"() -> (w439:string[][])
                                n296 = local write "Segments(s)"(w454) -> ()
                                n297 = call "RecordingDisplay_171213.vi"("TrackLength"=w435, "Segments"="DisplaySegments", "NormalMousebackgraound"=w452, "BackgroundSegments"=w451, "X"=w450, "Y"=w449, "i"="i", "X in"=w446, "Angle"=w434, "Y in"=w444) -> ("X out"=w445:i32[], "Y out"=w443:i32[], "RecordingDisplay"=→"RecordingDisplay":picture)  [unwired: 7 in]
                                n298 = local write "Current distance\n traveled (m)"(w455) -> ()
                                n299 = Add Array Elements(numeric array=w454) -> (sum=w453:dbl)
                                n300 = Increment(x="i") -> (x+1=w442:i32)
                                n301 = property on="Segements" class="Slide (strict)"("Scale.Maximum"=w453) -> ()  [unwired: 2 in, 2 out]
                                n302 = local write "i"(w442) -> ()
                                n303 = property on="SegmentsMulticolumnListbox" class="MCListbox (strict)"("ItemNames"=w439) -> ()  [unwired: 2 in, 2 out]
                                "Mouse speed (cm/s)" <- w457
                                "Mouse speed (cm/s)  2" <- w447
                                }
                              }
                              n304 = global read "Globaltracker.vi" "TrackerDisabled"() -> (w375:bool)
                              n305 = Or(x=w375, y="Stop Button") -> (x .or. y?=w366:bool)
                              n306 = global write "Globaltracker.vi" "Done"(w366) -> ()
                            }
                          }
                          frame True {
                            # "If the user wants to go back to settings before pressing start the program allows it in this way. Not recording means (pressing the Settings tab control ) to go to analysing page with those globals, which  immidietely sends the user back to the setting page \nand reset the parameters."
                            n307 = local read "Segments(s)"() -> (w458:dbl[])
                          }
                        }
                      }
                      frame #2 {
                        # "There would be an error to write some command to \nthe Tracker if it is not connected so there is a case\nstructure for this purpose."
                        n308 = case shown="False" w464 {
                          tunnel: w463 -> [w472 _]
                          tunnel: w462 -> [w471 _]
                          tunnel: w461 -> [w470 _]
                          frame False {
                            # "This saves the segments in the\nfolder in .bpm format."
                            n309 = local read "SegmentsRecalculation"() -> (w475:bool[])
                            n310 = local read "Mousebackground"() -> (w467:picture)
                            n311 = control-ref of="ProgressBar"() -> (w476:refnum<vi>)
                            n312 = call "LoadRecalcSave_171213.vi"("Segments"=w475, "Time"=w471, "Segments(s)"=w472, "LoadBackPath"=w470, "Slide in"=w476) -> ("ForAnalysisPath"=→"ForAnalysisLastRecordingPath":path, "ForSegmentsBMP"=w477:path)  [unwired: 5 in]
                            n313 = local write "Main TabControl"(enum32{"Settings", "Recording", "Analysis"}."Analysis" ("Main TabControl")) -> ()
                            n314 = call "Savingscreen_171213.vi"("NormalMouseBackgroundInput"=w467) -> ("Output"=w468:picture)  [unwired: 10 in]
                            n315 = invoke on="Loadedregions" class="Pict" method="Export Image"("File Type"=enum32{"BMP", "EPS", "EMF", "PICT"}."BMP", "Target"=enum32{"File", "Clipboard"}."File", "Path"=w477) -> ()  [unwired: 4 in, 7 out]
                            n316 = local write "AnalysisDisplay"(w468) -> ()
                          }
                          frame True {
                            # "If there was no recording, then there should\nnot be a saving procedure."
                          }
                        }
                        n317 = global read "Globaltracker.vi" "TrackerDisabled"() -> (w465:bool)
                        n318 = case shown="True" w465 {
                          selector: w465 -> [_ w484]
                          tunnel: w466 -> [w483 _]
                          frame False {
                            n319 = Concatenate Strings("O0" ("write buffer"), "\r") -> (w480:string)
                            n320 = VISA Write(VISA resource name=w483, write buffer=w480) -> (VISA resource name out=w479:refnum<visa-resource-name>)  [unwired: 1 in, 2 out]
                            n321 = VISA Close(VISA resource name=w479) -> ()  [unwired: 1 in, 1 out]
                          }
                          frame True {
                            n322 = global write "Globaltracker.vi" "Analysiss"(w484) -> ()
                          }
                        }
                      }
                    }
                  }
                  frame True {
                    # "An error window comes on the screen and tells the problem : The tracker is not connected. After the okay button pressed the program goes to the analysing part\nbecause that is the only thing what a user can do without the tracker."
                    n323 = global write "Globaltracker.vi" "Analysiss"(w485) -> ()
                    n324 = flat-sequence {
                      frame #0 {
                        n325 = One Button Dialog(message="ERROR:Tracker is not connected") -> ()  [unwired: 1 in, 1 out]
                      }
                      frame #1 {
                        n326 = local write "Main TabControl"(enum32{"Settings", "Recording", "Analysis"}."Analysis" ("Main TabControl")) -> ()
                      }
                    }
                  }
                }
              }
              frame True {
                # "If analysis was clicked by the user the program skips the recording part"
                n327 = local write "LOAD RECORDING"(FALSE ("LOAD")) -> ()
              }
            }
          }
          frame #2 {
            # "Analysis tab of main screen"
            n328 = global read "Globaltracker.vi" "Analysiss"() -> (w489:bool)
            n329 = case shown="True" w489 {
              frame False {
                n330 = local write "LOAD RECORDING"(TRUE ("LOAD RECORDING")) -> ()
              }
              frame True {
                n331 = local write "LOAD RECORDING"(FALSE ("LOAD")) -> ()
              }
            }
            n332 = while {
              tunnel: ["EXIT"] -> w490
              tunnel: w489 -> [_]
              stop <- w494 stop-if-true
              # "This is the main loop in the analyzis part. This allows to analyze multiple files until the user exits the program or goes back to setting for a new recording,"
              n333 = case shown="True" "LOAD RECORDING" {
                tunnel: [w499 w516] -> w496
                frame False {
                  w497 = FALSE ("Stop Button 2")
                  w498 = 0.0 ("SUM PATH ( m) 2")
                  w505 = "" ("date/time string A")
                  # "In this case while the program waits for the user to load in a recording. It displays Load a Recording on the canvas. Make all the variables back to default.\nAnd let the user go back to the fistt page ( settings) to make a new recording ( after saving the settings )"
                  n334 = local read "Mousebackground"() -> (w504:picture)
                  n335 = local write "FileName"(w505) -> ()
                  n336 = local write "Mouse Speed plotted vs time"(w498) -> ()
                  n337 = global write "Globaltracker.vi" "CounterDownforPlaybackSpeed"(w498) -> ()
                  n338 = global write "Globaltracker.vi" "CounterUpforPlaybackSpeed"(w498) -> ()
                  n339 = local write "Current Distance\n Traveled (m)"(w498) -> ()
                  n340 = local write "Playback progress (min)"(w498) -> ()
                  n341 = local write "Playback progress (min)"(w498) -> ()
                  n342 = local write "Total Distance Traveled (m)"(w498) -> ()
                  n343 = local write "Mouse speed (cm/s)"(w498) -> ()
                  n344 = local write "Average Speed (cm/s)"(w498) -> ()
                  n345 = local write "Display Speed"(w498) -> ()
                  n346 = local write "index"(w498) -> ()
                  n347 = local write "date/time"(w505) -> ()
                  n348 = property on="Playback progress (min)" class="Slide (strict)"("Scale.Minimum"=w498) -> ()  [unwired: 2 in, 2 out]
                  n349 = property on="Mouse Speed plotted vs time" class="WFChart (strict)"("History Data"=dbl[] []) -> ()  [unwired: 2 in, 2 out]
                  n350 = call "LoadRecordingscreen_171213.vi"("Input"=w504) -> ("Output"=w503:picture)  [unwired: 10 in]
                  n351 = local write "AnalysisDisplay"(w503) -> ()
                  n352 = local write "Seek Forward Button"(w497) -> ()
                  n353 = global write "Globaltracker.vi" "TrackerDisabled"(w497) -> ()
                  n354 = local write "Skip Forward Button"(w497) -> ()
                  n355 = local write "Seek Back Button"(w497) -> ()
                  n356 = local write "Stop Button"(w497) -> ()
                  n357 = local write "Heat Map"(w497) -> ()
                  n358 = local write "RemoveButton"(w497) -> ()
                  n359 = local write "SegmentsOn"(w497) -> ()
                  n360 = local write "Skip Back Button"(w497) -> ()
                  n361 = local write "AddButton"(w497) -> ()
                  n362 = local write "FullTrack"(w497) -> ()
                  n363 = local read "Main TabControl"() -> (w502:enum32{"Settings", "Recording", "Analysis"})
                  n364 = Equal?(x=w502, y=enum32{"Setting", "Recording", "Analysis"}."Setting") -> (x = y?=w501:bool)
                  n365 = case shown="True" w501 {
                    selector: w501 -> [_ w508]
                    tunnel: [FALSE w508] -> w499
                    frame False {
                    }
                    frame True {
                      w509 = FALSE ("HTrackerOff")
                      n366 = global write "Globaltracker.vi" "Analysiss"(w509) -> ()
                      n367 = local write "SAVE"(w509) -> ()
                    }
                  }
                }
                frame True {
                  # "If the user select a file the analyzis steps forward\nif it is cancelled or closes then the analyzing part\nis skipped and the program goes to the waiting\nstate where the new decision can be made by \nthe user. Load another one, exit , or go to setting\nand record a new one."
                  # "This starts also with a case structure because\nidially the program immedietaly loads back \nthe last recording. If it is not the last recording \nthen it waits for the user to select a file."
                  # "This case structure allows to reload or wait for an another decision like exit or new recording or load an other recording"
                  n368 = global read "Globaltracker.vi" "Analysiss"() -> (w514:bool)
                  n369 = Not(x=w514) -> (.not. x?=w515:bool)
                  n370 = case shown="True" w515 {
                    tunnel: [w521 w523] -> w511
                    tunnel: [w517 FALSE ("cancelled")] -> w513
                    frame False {
                      n371 = call "File Dialog"() -> ("selected path"=w521:path, "cancelled"=w518:bool, "error out"=w520:errorcluster)  [unwired: 12 in, 1 out]
                      n372 = Unbundle(w520) -> ("status"=w519:bool)  [unwired: 2 out]
                      n373 = Or(x=w519, y=w518) -> (x .or. y?=w517:bool)
                    }
                    frame True {
                      n374 = local read "ForAnalysisLastRecordingPath"() -> (w523:path)
                    }
                  }
                  n375 = Not(x=w513) -> (.not. x?=w512:bool)
                  n376 = local write "LOAD RECORDING"(w512) -> ()
                  n377 = case shown="True" w512 {
                    tunnel: [FALSE w543] -> w516
                    tunnel: w513 -> [_ w539]
                    tunnel: w511 -> [_ w541]
                    frame False {
                      # "The program goes back to the waiting state:  where the new decision can be made by \nthe user. Load another one, exit , or go to setting and record a new one."
                    }
                    frame True {
                      w525 = FALSE ("Stop Button 2")
                      w528 = 0.0 ("SUM PATH ( m) 2")
                      # "This case structure is the analyzing part before entering a loop the actual playback. It starts with calculation outside of the loop to let the loop run on max iteration speed. And sets the values back to default."
                      n378 = local read "Mousebackground"() -> (w526:picture)
                      n379 = call "ReloadCSVforanalysispart_171213.vi"("Path"=w541) -> ("Clean data array"=w538:dbl[][], "Time"=w542:string[])  [unwired: 1 in, 3 out]
                      n380 = call "LoadFileName_171213.vi"("SelectedPath"=w541) -> ("FIleName"=→"FileName":string)  [unwired: 10 in]
                      n381 = call "Transformationto360x360matrixcoordinates_171213.vi"("FilteredInputData"=w538) -> ("360Y"=w534:dbl[], "360X"=w535:dbl[])  [unwired: 9 in]
                      n382 = local write "Start/play"(w525) -> ()
                      n383 = property on="Playback progress (min)" class="Slide (strict)"("Scale.Minimum"=w528) -> ()  [unwired: 2 in, 2 out]
                      n384 = local write "Seek Forward Button"(w525) -> ()
                      n385 = local write "LOAD RECORDING"(w525) -> ()
                      n386 = local write "Skip Forward Button"(w525) -> ()
                      n387 = global write "Globaltracker.vi" "CounterDownforPlaybackSpeed"(w528) -> ()
                      n388 = global write "Globaltracker.vi" "CounterUpforPlaybackSpeed"(w528) -> ()
                      n389 = local write "Seek Back Button"(w525) -> ()
                      n390 = local write "Stop Button"(w525) -> ()
                      n391 = local write "Heat Map"(w525) -> ()
                      n392 = local write "Skip Back Button"(w525) -> ()
                      n393 = local write "SegmentsOn"(w525) -> ()
                      n394 = local write "RemoveButton"(w525) -> ()
                      n395 = local write "Playback progress (min)"(w528) -> ()
                      n396 = local write "AddButton"(w525) -> ()
                      n397 = local write "FullTrack"(w525) -> ()
                      n398 = local write "FullTrack"(w525) -> ()
                      n399 = property on="Current Distance Traveled (m)" class="Slide (strict)"("Scale.Minimum"=w528) -> ()  [unwired: 2 in, 2 out]
                      n400 = case shown="False" w539 {
                        tunnel: w526 -> [w545 w547]
                        tunnel: [w544 w546] -> w540
                        frame False {
                          n401 = call "Loadingscreen_171213.vi"("2D Picture"=w545) -> ("2D Picture 2"=w544:picture)  [unwired: 10 in]
                        }
                        frame True {
                          n402 = call "LoadRecordingscreen_171213.vi"("Input"=w547) -> ("Output"=w546:picture)  [unwired: 10 in]
                        }
                      }
                      n403 = control-ref of="ProgressBar"() -> (w537:refnum<vi>)
                      n404 = local write "Playback Speed"("1 X" ("Display Speed")) -> ()
                      n405 = call "BackgroundFulltrackCalculations_171213.vi"("360Y"=w534, "Mousebackground"=w526, "360X"=w535, "ForAnalysisLastRecordingPath"=w541, "Slide in"=w537) -> ("BackgroundSegmentforAnalysis"=w536:picture, "NormalMousebackgroundOutput"=w532:picture, "BackgroundSegmentsOutput"=w533:picture, "HeatMap"=→"Heat-Map":dbl[][])  [unwired: 3 in]
                      n406 = local write "AnalysisDisplay"(w540) -> ()
                      n407 = while {
                        tunnel: [FALSE] -> w543
                        tunnel: w538 -> [w564]
                        tunnel: w542 -> [w563]
                        tunnel: w536 -> [w562]
                        tunnel: w534 -> [w561]
                        tunnel: w535 -> [w560]
                        tunnel: w533 -> [w559]
                        tunnel: w532 -> [w558]
                        tunnel: w526 -> [w554]
                        stop <- w557 stop-if-true
                        # "This loop is the analyzing the same file over and over again until the user does not say new file or exists the program or goes back for and other recording."
                        n408 = flat-sequence {
                          tunnel: [w592] -> w572
                          tunnel: [w591] -> w570
                          tunnel: [w590] -> w571
                          tunnel: [w589] -> w569
                          tunnel: [w588] -> w568
                          tunnel: [w587] -> w567
                          tunnel: [w574] -> w566
                          tunnel: w563 -> [w592]
                          tunnel: w562 -> [w591]
                          tunnel: w561 -> [w590]
                          tunnel: w560 -> [w574]
                          tunnel: w564 -> [w577]
                          tunnel: w554 -> [w589]
                          tunnel: w558 -> [w588]
                          tunnel: w559 -> [w587]
                          tunnel: [w585] -> w553
                          tunnel: [w580] -> w552
                          tunnel: [w579] -> w551
                          tunnel: [w578] -> w550
                          tunnel: [i32[] [] ("Y out 5")] -> w549
                          tunnel: [w573] -> w548
                          tunnel: w572 -> [w611]
                          tunnel: w571 -> [w610]
                          tunnel: w570 -> [w609]
                          tunnel: w569 -> [w608]
                          tunnel: w568 -> [w606]
                          tunnel: w567 -> [w607]
                          tunnel: w566 -> [w605]
                          tunnel: [w604] -> w555
                          tunnel: w553 -> [w603]
                          tunnel: w552 -> [w602]
                          tunnel: w551 -> [w601]
                          tunnel: w550 -> [w600]
                          tunnel: w549 -> [w599]
                          tunnel: w548 -> [w598]
                          tunnel: [w760] -> w556
                          tunnel: w555 -> [w760]
                          tunnel: [w765] -> w557
                          tunnel: w556 -> [w764]
                          frame #0 {
                            # "This frame waits for the user to \npress the start button.\nIt displays the constant vaules or sets\nback to default."
                            n409 = call "SumTimeSpendAnalyze_171213.vi"("Clean data array"=w577) -> ("Item Names"=w586:string[][])  [unwired: 10 in]
                            n410 = while {
                              stop <- w595 stop-if-true
                              n411 = local read "Mousebackground"() -> (w597:picture)
                              n412 = local read "EXIT"() -> (w593:bool)
                              n413 = Or(x="Start/play", y=w593) -> (x .or. y?=w595:bool)
                              n414 = call "PressPlay_171213.vi"("Input"=w597) -> ("Output"=w596:picture)  [unwired: 10 in]
                              n415 = local write "AnalysisDisplay"(w596) -> ()
                            }
                            n416 = property on="TimeSpentinEachSegmentMultiListBox" class="MCListbox (strict)"("ItemNames"=w586) -> ()  [unwired: 2 in, 2 out]
                            n417 = property on="Mouse Speed plotted vs time" class="WFChart (strict)"("History Data"=dbl[] []) -> ()  [unwired: 2 in, 2 out]
                            n418 = call "SelectColumnstoPlaybackDisplay_171213.vi"("Clean data array in"=w577) -> ("Speed"=w585:dbl[], "TotalDIstanceTraveled"=w584:dbl, "Playbackprogress(min)maxscale"=w583:dbl, "CurrentDIstancemaxScale"=w582:dbl, "AVGSpeed"=w581:dbl, "CurrentDistanceTraveled"=w580:dbl[], "TTL"=w579:dbl[], "Angle"=w578:dbl[])  [unwired: 3 in]
                            n419 = property on="Playback progress (min)" class="Slide (strict)"("Scale.Maximum"=w583) -> ()  [unwired: 2 in, 2 out]
                            n420 = local write "Total Distance Traveled (m)"(w584) -> ()
                            n421 = local write "Average Speed (cm/s)"(w581) -> ()
                            n422 = property on="Current Distance\n Traveled (m)" class="Slide (strict)"("Scale.Maximum"=w582) -> ()  [unwired: 2 in, 2 out]
                            n423 = Array Size(array=w574) -> (size(s)=w573:i32)
                          }
                          frame #1 {
                            n424 = while {
                              tunnel: w609 -> [w649]
                              shift-right: [w648] -> _
                              shift-left: w599 -> [w647]
                              shift-right: [w646] -> _
                              shift-left: w599 -> [w645]
                              tunnel: w598 -> [w613]
                              tunnel: w611 -> [w621]
                              tunnel: w610 -> [w636]
                              tunnel: w605 -> [w635]
                              tunnel: w608 -> [w620]
                              tunnel: w607 -> [w615]
                              tunnel: w606 -> [w617]
                              tunnel: [w628] -> w604
                              tunnel: w603 -> [w627]
                              tunnel: w602 -> [w626]
                              tunnel: w601 -> [w624]
                              tunnel: w600 -> [w625]
                              stop <- w629 stop-if-true
                              # "This loop is responsible for the analyzing display"
                              n425 = flat-sequence {
                                tunnel: [w668] -> w644
                                tunnel: [w667] -> w643
                                tunnel: [w666] -> w642
                                tunnel: [w659] -> w641
                                tunnel: [w657] -> w640
                                tunnel: [w661] -> w639
                                tunnel: [w662] -> w638
                                tunnel: w649 -> [w668]
                                tunnel: w647 -> [w667]
                                tunnel: w645 -> [w666]
                                tunnel: [w658] -> w637
                                tunnel: w636 -> [w662]
                                tunnel: w635 -> [w661]
                                tunnel: w627 -> [w659]
                                tunnel: w626 -> [w658]
                                tunnel: w625 -> [w657]
                                tunnel: w624 -> [w656]
                                tunnel: [w656] -> w623
                                tunnel: [w655] -> w622
                                tunnel: w621 -> [w655]
                                tunnel: w620 -> [w654]
                                tunnel: [w654] -> w619
                                tunnel: [w653] -> w618
                                tunnel: w617 -> [w653]
                                tunnel: [w652] -> w616
                                tunnel: w615 -> [w652]
                                tunnel: [w651] -> w614
                                tunnel: w613 -> [w651]
                                tunnel: [w696] -> w628
                                tunnel: w644 -> [w731]
                                tunnel: w643 -> [w730]
                                tunnel: w642 -> [w729]
                                tunnel: w641 -> [w727]
                                tunnel: w640 -> [w726]
                                tunnel: w639 -> [w724]
                                tunnel: w638 -> [w722]
                                tunnel: w637 -> [w720]
                                tunnel: [w709] -> w634
                                tunnel: [w707] -> w632
                                tunnel: w623 -> [w683]
                                tunnel: w622 -> [w682]
                                tunnel: w619 -> [w681]
                                tunnel: w618 -> [w680]
                                tunnel: w616 -> [w679]
                                tunnel: w614 -> [w678]
                                tunnel: [w670] -> w612
                                tunnel: w634 -> [w751]
                                tunnel: [w751] -> w633
                                tunnel: w632 -> [w750]
                                tunnel: [w750] -> w631
                                tunnel: w612 -> [w748]
                                tunnel: [w757] -> w648
                                tunnel: [w758] -> w646
                                tunnel: w633 -> [w757]
                                tunnel: w631 -> [w758]
                                frame #0 {
                                n426 = Multiply(x="Playback progress (min)", y=60.0) -> (x*y=w663:dbl)
                                n427 = Multiply(x=w663, y=80) -> (x*y=w650:dbl)
                                n428 = global write "Globaltracker.vi" "index"(w650) -> ()
                                }
                                frame #1 {
                                n429 = global read "Globaltracker.vi" "index"() -> (w669:i16)
                                n430 = case shown="False" "Heat Map" {
                                frame False {
                                n431 = flat-sequence {
                                frame #0 {
                                n432 = property on="AnalysisDisplay" class="Pict"("Visible"=TRUE) -> ()  [unwired: 2 in, 2 out]
                                }
                                frame #1 {
                                n433 = property on="Heat-Map" class="IntGraph (strict)"("Visible"=FALSE) -> ()  [unwired: 2 in, 2 out]
                                }
                                }
                                }
                                frame True {
                                n434 = flat-sequence {
                                frame #0 {
                                n435 = property on="Heat-Map" class="IntGraph (strict)"("Visible"=TRUE) -> ()  [unwired: 2 in, 2 out]
                                }
                                frame #1 {
                                n436 = property on="AnalysisDisplay" class="Pict"("Visible"=FALSE) -> ()  [unwired: 2 in, 2 out]
                                }
                                }
                                }
                                }
                                n437 = Index Array(array=w720, index=w669) -> (element=w719:dbl)
                                n438 = Index Array(array=w727, index=w669) -> (element=w703:dbl)
                                n439 = Index Array(array=w682, index=w669) -> (element=w702:string)
                                n440 = Index Array(array=w683, index=w669) -> (element=w699:dbl)
                                n441 = Index Array(array=w726, index=w669) -> (element=w725:dbl)
                                n442 = Index Array(array=w724, index=w669) -> (element=w723:dbl)
                                n443 = Index Array(array=w722, index=w669) -> (element=w721:dbl)
                                n444 = local write "Mouse Speed plotted vs time"(w703) -> ()
                                n445 = local write "Current Distance\n Traveled (m)"(w719) -> ()
                                n446 = local write "Mouse speed (cm/s)"(w703) -> ()
                                n447 = local write "date/time"(w702) -> ()
                                n448 = Equal?(x=1.0, y=w699) -> (x = y?=→"TTL":bool)
                                n449 = Multiply(x="Trace_length (s)", y=80.0) -> (x*y=w733:dbl)
                                n450 = Round To Nearest(number=w733) -> (nearest integer value=w728:dbl)
                                n451 = Increment(x=w669) -> (x+1=w677:i16)
                                n452 = call "AnalysisDisplay_171213.vi"("TraceLength"=w728, "Segments"="SegmentsOn", "FullTrack"="FullTrack", "FulltrackonBackgroundSegments"=w679, "BackgroundSegments"=w731, "NormalMouseBackground"=w681, "X"=w723, "Y"=w721, "i"=w677, "X in"=w730, "Angle"=w725, "Y in"=w729, "FulltrackonNormalMouseBackground"=w680) -> ("X out"=w716:i32[], "Y out"=w715:i32[], "AnalysisDisplayOutput"=→"AnalysisDisplay":picture)  [unwired: 4 in]
                                n453 = global write "Globaltracker.vi" "index"(w677) -> ()
                                n454 = Or(x="Skip Forward Button", y="Skip Back Button") -> (x .or. y?=w706:bool)
                                n455 = Or(x="Seek Forward Button", y="Seek Back Button") -> (x .or. y?=w705:bool)
                                n456 = Add(x=w669, y=400) -> (x+y=w717:i32)
                                n457 = Or(x=w706, y=w705) -> (x .or. y?=w704:bool)
                                n458 = Greater Or Equal?(x=w669, y=w678) -> (x >= y?=w700:bool)
                                n459 = control-ref of="Skip Back Button"() -> (w674:refnum<vi>)
                                n460 = call "Skipback_171213.vi"("Y out 3"=w715, "X in"=w716, "Skip Back Button"="Skip Back Button", "Boolean in"=w674) -> ("Y out"=w713:i32[], "Y out 2"=w714:i32[])  [unwired: 6 in]
                                n461 = case shown="True" w704 {
                                tunnel: w669 -> [_ w743]
                                tunnel: w717 -> [_ w742]
                                frame False {
                                # "This Case straucture is only for the Mouse Speed \nplotted vs Time display. Especially the scale and \nmemory of that indicator. \nIf the users changes time position of the playback\nby using the playback buttons, then the memory of\nthis display indicator is cleared."
                                }
                                frame True {
                                n462 = flat-sequence {
                                tunnel: w743 -> [w746]
                                tunnel: w742 -> [w745]
                                frame #0 {
                                n463 = property on="Mouse Speed plotted vs time" class="WFChart (strict)"("History Data"=dbl[] []) -> ()  [unwired: 2 in, 2 out]
                                }
                                frame #1 {
                                n464 = property on="Mouse Speed plotted vs time" class="WFChart (strict)"("XScale.Maximum"=w745, "XScale.Minimum"=w746) -> ()  [unwired: 2 in, 2 out]
                                }
                                }
                                }
                                }
                                n465 = event shown="[1] \"AddButton\": Mouse Down" {
                                selector: _ -> [_ _ _]
                                dyn-events: _ -> [_ _ _]
                                timeout: 0 -> [_ _ _]
                                event Timeout {
                                n466 = event-data() -> ()  [unwired: 1 in, 3 out]
                                }
                                event "AddButton": Mouse Down {
                                n467 = event-data() -> ()  [unwired: 1 in, 2 out]
                                n468 = global read "Globaltracker.vi" "CounterUpforPlaybackSpeed"() -> (w734:i16)
                                n469 = Increment(x=w734) -> (x+1=w735:i16)
                                n470 = global write "Globaltracker.vi" "CounterUpforPlaybackSpeed"(w735) -> ()
                                }
                                event "RemoveButton": Mouse Down {
                                n471 = event-data() -> ()  [unwired: 1 in, 1 out]
                                n472 = global read "Globaltracker.vi" "CounterDownforPlaybackSpeed"() -> (w736:i16)
                                n473 = Increment(x=w736) -> (x+1=w737:i16)
                                n474 = global write "Globaltracker.vi" "CounterDownforPlaybackSpeed"(w737) -> ()
                                }
                                }
                                n475 = control-ref of="Skip Forward Button"() -> (w673:refnum<vi>)
                                n476 = call "Skipforward_171213.vi"("Y out 3"=w713, "Y out 4"=w714, "Skip Forward Button"="Skip Forward Button", "Boolean in"=w673) -> ("Y out"=w711:i32[], "Y out 2"=w712:i32[])  [unwired: 6 in]
                                n477 = local read "Start/play"() -> (w694:bool)
                                n478 = local read "EXIT"() -> (w675:bool)
                                n479 = Or(x="Stop Button", y=w700) -> (x .or. y?=w696:bool)
                                n480 = Or(x=w694, y=w675) -> (x .or. y?=w693:bool)
                                n481 = control-ref of="Seek Back Button"() -> (w672:refnum<vi>)
                                n482 = call "SeekBack_171213.vi"("Y out 3"=w711, "Y out 4"=w712, "Seek Back Button"="Seek Back Button", "Boolean in"=w672) -> ("Y out"=w708:i32[], "Y out 2"=w710:i32[])  [unwired: 6 in]
                                n483 = call "Displayspeed_171213.vi"() -> ("DisplaySpeed"=w670:dbl, "Waitin(ms)"=w701:dbl)  [unwired: 10 in]
                                n484 = case shown="False" w693 {
                                frame False {
                                n485 = while {
                                stop <- w747 stop-if-true
                                n486 = local read "Start/play"() -> (w747:bool)
                                }
                                }
                                frame True {
                                }
                                }
                                n487 = Wait (ms)(milliseconds to wait=w701) -> ()  [unwired: 1 out]
                                n488 = control-ref of="Seek Forward Button"() -> (w671:refnum<vi>)
                                n489 = call "SeekForward_171213.vi"("Y in"=w708, "Y out 4"=w710, "Seek Forward Button"="Seek Forward Button", "Boolean in"=w671) -> ("Y out"=w707:i32[], "Y out 3"=w709:i32[])  [unwired: 6 in]
                                }
                                frame #2 {
                                n490 = call "DisplaySpeedDisplay_171213.vi"("Display Speed"=w748) -> ("PlayBackSpeedDisplay"=→"Playback Speed":string)  [unwired: 10 in]
                                n491 = call "IndexCheckifBelow0_171213.vi"() -> ()  [unwired: 12 in]
                                }
                                frame #3 {
                                n492 = global read "Globaltracker.vi" "index"() -> (w752:i16)
                                n493 = Divide(x=w752, y=80.0) -> (x/y=w754:dbl)
                                n494 = Divide(x=w754, y=60.0) -> (x/y=w756:dbl)
                                n495 = local write "Playback progress (min)"(w756) -> ()
                                }
                              }
                              n496 = local read "EXIT"() -> (w630:bool)
                              n497 = Or(x=w628, y=w630) -> (x .or. y?=w629:bool)
                            }
                          }
                          frame #2 {
                            w759 = 0 ("index")
                            w762 = FALSE
                            n498 = local read "Mousebackground"() -> (w763:picture)
                            n499 = local write "AnalysisDisplay"(w763) -> ()
                            n500 = local write "ProgressBar"(w759) -> ()
                            n501 = local write "Stop Button"(w762) -> ()
                            n502 = local write "Start/play"(w762) -> ()
                            n503 = global write "Globaltracker.vi" "Analysiss"(TRUE ("Anal")) -> ()
                            n504 = global write "Globaltracker.vi" "index"(w759) -> ()
                          }
                          frame #3 {
                            n505 = local read "EXIT"() -> (w766:bool)
                            n506 = case shown="False" w766 {
                              selector: w766 -> [_ w777]
                              tunnel: w764 -> [w768 _]
                              tunnel: [w767 w777] -> w765
                              frame False {
                                n507 = case shown="True" w768 {
                                tunnel: [w769 w773] -> w767
                                frame False {
                                n508 = Two Button Dialog(message="Do you want to load a new recording?", 1:"No" ("F button name (\"Cancel\")"), 2:"Yes" ("T button name (\"OK\")")) -> (T button?=w769:bool)
                                }
                                frame True {
                                n509 = Two Button Dialog(message="Do you want to load a new recording?", 1:"No" ("F button name (\"Cancel\")"), 2:"Yes" ("T button name (\"OK\")")) -> (T button?=w773:bool)
                                }
                                }
                              }
                              frame True {
                              }
                            }
                          }
                        }
                      }
                      "Current Distance\n Traveled (m)" <- w528
                      "Mouse speed (cm/s)" <- w528
                      "Mouse Speed plotted vs time" <- w528
                      "Average Speed (cm/s)" <- w528
                      "Total Distance Traveled (m)" <- w528
                      "Display Speed" <- w528
                      "index" <- w528
                      "date/time" <- "" ("date/time string 2")
                    }
                  }
                  "ProgressBar" <- u16 0 ("ProgressBar")
                }
              }
              n510 = Or(x=w496, y="EXIT") -> (x .or. y?=w494:bool)
            }
          }
        }
      }
    }
  }
  n511 = disable-structure shown="Enabled" {
    frame Disabled {
      n512 = Seconds To Date/Time() -> (date time rec=w785:T9)  [unwired: 2 in]
      n513 = Unbundle By Name(w785) -> ("fractional second"=w784:dbl, "second"=w783:i32, "minute"=w782:i32, "hour"=w781:i32)
      n514 = formula code="S=ms+s;\nM=S/60+m;\nH=M/60+h;"("ms"=w784, "s"=w783, "m"=w782, "h"=w781) -> ("M"=w780:dbl, "H"=w779:dbl, "S"=w778:dbl)
      n515 = Bundle("M"=w780, "H"=w779, "S"=w778) -> ()  [unwired: 1 in, 1 out]
    }
    frame Enabled {
    }
  }
